vi "Lockin-4461_Multiple Inputs and Outputs_KH.vi"(8 "stop":bool) -> (3 "Input signal":dbl[][](graph))   [LabVIEW 2013]
uses:
  <vilib>/DAQmx/write.llb/DAQmx Write (Analog 1D Wfm NChan NSamp).vi
  DAQ-Lockin-SubVI/Lock-in Globles Multiple Inputs and Outputs used with FGV.vi
  DAQ-Lockin-SubVI/Lock-in Globles Multiple Inputs and Outputs.vi
  <vilib>/DAQmx/miscellaneous.llb/DAQmx Fill In Error Info.vi
  Q:/inst/Leiden measurements VIs/IV measurement/Sub VIs/Global Value.vi
  <vilib>/Analysis/NI_AALPro.lvlib
  <vilib>/Analysis/2dsp.llb/Decimate (single shot, DBL).vi
panel:
  out "Data":waveform(dbl)[][](array[waveform])=[[{"t0"=timestamp(0 s since 1904-01-01), "dt"=5.17729651930355e-06, "Y"=array[14350 elements]}, {"t0"=timestamp(0 s since 1904-01-01), "dt"=5.17729651930355e-06, "Y"=array[14350 elements]}], [{"t0"=timestamp(0 s since 1904-01-01), "dt"=5.17729651930355e-06, "Y"=array[14350 elements]}, {"t0"=timestamp(0 s since 1904-01-01), "dt"=5.17729651930355e-06, "Y"=array[14350 elements]}], [{"t0"=timestamp(0 s since 1904-01-01), "dt"=5.17729651930355e-06, "Y"=array[14350 elements]}, {"t0"=timestamp(0 s since 1904-01-01), "dt"=5.17729651930355e-06, "Y"=array[14350 elements]}], [{"t0"=timestamp(0 s since 1904-01-01), "dt"=5.17729651930355e-06, "Y"=array[14350 elements]}, {"t0"=timestamp(0 s since 1904-01-01), "dt"=5.17729651930355e-06, "Y"=array[14350 elements]}]]
  out "phase log":dbl[](array[numeric])=[0.9999999998974775, 0.9999999998974775, 0.9999999998974775, 0.9999999998974775]
  in  "Tab Control 2":T1(tab)=enum."Lock-in Settings"
  in  "max ai rate":i32=200000
  in  "Auto control  max AI rate/ AI block size":bool=TRUE
  in  "AI Buffer Size (s)":i32=10
  in  "AI Block Size":i32=14350
  out "AI Rate":dbl=193151.0 format="%.2f"
  in  "AI Configuration":T2(array[cluster])=[{"AI.Coupling"=10050, "AI.Max"=10.0, "AI.Min"=-10.0, "Input physical channels"="PXI1Slot2/ai0:1"}, {"AI.Coupling"=10050, "AI.Max"=10.0, "AI.Min"=-10.0, "Input physical channels"="PXI1Slot3/ai0:1"}, {"AI.Coupling"=10050, "AI.Max"=10.0, "AI.Min"=-10.0, "Input physical channels"="PXI1Slot5/ai0:1"}, {"AI.Coupling"=10050, "AI.Max"=10.0, "AI.Min"=-10.0, "Input physical channels"="PXI1Slot6/ai0:1"}] {"AI.Coupling" items=["AC"=10045, "DC"=10050, "GND"=10066]}
  in  "AO Configuration":T3(array[cluster])=[{"Output physical channels"="PXI1Slot2/ao0:1", "AO. Max"=0.1, "AO.Min"=-0.1}, {"Output physical channels"="PXI1Slot3/ao0:1", "AO. Max"=0.25, "AO.Min"=-0.25}, {"Output physical channels"="PXI1Slot5/ao0:1", "AO. Max"=0.1, "AO.Min"=-0.1}, {"Output physical channels"="PXI1Slot6/ao0:1", "AO. Max"=0.1, "AO.Min"=-0.1}]
  in  "OSC Configuration":T4(array[cluster])=[[{"Signal Type"=enum."Sine Wave", "DC"=0.0, "Amplitude"=0.0, "frequency"=13.46, "Phase"=0.0}, {"Signal Type"=enum."Sine Wave", "DC"=0.0, "Amplitude"=0.0005, "frequency"=13.46, "Phase"=0.0}], [{"Signal Type"=enum."Sine Wave", "DC"=0.0, "Amplitude"=0.0, "frequency"=13.46, "Phase"=0.0}, {"Signal Type"=enum."Sine Wave", "DC"=0.0, "Amplitude"=0.0, "frequency"=13.46, "Phase"=0.0}], [{"Signal Type"=enum."Sine Wave", "DC"=0.0, "Amplitude"=0.0, "frequency"=13.46, "Phase"=0.0}, {"Signal Type"=enum."Sine Wave", "DC"=0.0, "Amplitude"=0.0, "frequency"=13.46, "Phase"=0.0}], [{"Signal Type"=enum."Sine Wave", "DC"=-0.0467, "Amplitude"=0.0, "frequency"=13.46, "Phase"=0.0}, {"Signal Type"=enum."Sine Wave", "DC"=0.0, "Amplitude"=0.0, "frequency"=13.46, "Phase"=0.0}]] {"frequency" step=0.001 format="%.3p"; "Amplitude" format="%0.2p"; "DC" min=-0.99 max=0.99 format="%.2p"}
  in  "Phase&Tc":T5(array[cluster])=[{"Phase"=0.0, "Time constant"=0.5, "Set Tc"=FALSE, "Autophase"=FALSE, "Order"=0.0}, {"Phase"=0.0, "Time constant"=0.5, "Set Tc"=FALSE, "Autophase"=FALSE, "Order"=0.0}, {"Phase"=0.0, "Time constant"=0.5, "Set Tc"=FALSE, "Autophase"=FALSE, "Order"=0.0}, {"Phase"=0.0, "Time constant"=0.5, "Set Tc"=FALSE, "Autophase"=FALSE, "Order"=0.0}, {"Phase"=0.0, "Time constant"=0.5, "Set Tc"=FALSE, "Autophase"=FALSE, "Order"=0.0}, {"Phase"=0.0, "Time constant"=0.5, "Set Tc"=FALSE, "Autophase"=FALSE, "Order"=0.0}, {"Phase"=0.0, "Time constant"=0.5, "Set Tc"=FALSE, "Autophase"=FALSE, "Order"=0.0}, {"Phase"=0.0, "Time constant"=0.5, "Set Tc"=FALSE, "Autophase"=FALSE, "Order"=0.0}] {"Phase" min=0.0 max=360.0 scale=0.0..360.0}
  out "Gain":dbl[](array[numeric])=[0.001, 2e-08, 0.001, 0.001, 0.001, 2e-08]
  out "Display 2":string="-189.706780      pA"
  out "Display 1":string="-  1.195069      nA"
  in  "Remote":bool=TRUE
  in  "Display":u16(ring) items=["X and Y", "R and Theta"]
  out "Results":dbl[][](array[numeric])=[[0.0009525094408010766, 3.177938793839466e-05, 0.0009530394348152224, 1.910899317245332], [-0.05975347202365848, -0.009485339009678177, 0.060501645225652, -170.98005941712123], [-3.4755069590434e-06, 9.053140207140873e-07, 3.591481880569719e-06, 165.3998106146712], [0.3512155559510749, -0.06667061103568536, 0.3574875342132845, -10.748465433064244], [0.014508685424842276, -0.002760839766845655, 0.014769028030822714, -10.773934547991182], [0.017218857649450085, -0.002713178173891731, 0.017431305015841704, -8.954481243481103], [-1.0027706515450597e-06, 6.692232605674919e-07, 1.2055740342611434e-06, 146.2818764335927], [-1.3255838707835008e-06, -9.034329256038387e-07, 1.6041707046154658e-06, -145.72416746774206]]
  out "Backlog":u8(slide) scale=0.0..100.0
  out "Sampling information":cluster{"Fs":dbl, "#s":dbl}[](array[cluster])=[{"Fs"=193151.0, "#s"=14350.0}, {"Fs"=193151.0, "#s"=14350.0}, {"Fs"=193151.0, "#s"=14350.0}, {"Fs"=193151.0, "#s"=14350.0}]
  out "AO Task":refnum<k21>[](array[refnum])
  out "AI task":refnum<k21>[](array[refnum])
  out "Signal":dbl[][](array[numeric])
  in  "Tab Control":T6(tab)=enum."Input signals"
  in  "Lockin Display A":i16(slide)=4 scale=1.0..18.0
  out "Display X (or R) A":dbl[](graph)=[0.0003515597766155211, 0.0003507181675748926, 0.00035141371795365553, 0.0003511676429896116, 0.00035187230028368424, 0.00035142951363845783, 0.00035200218342147584, 0.0003516475669745772, 0.0003513264804061819, 0.0003512466291338144, 0.00035057064868592705, 0.0003509796679868739, 0.0003503537452691344, 0.00035135722504198624, 0.0003499281739531895, 0.00035086727974118317, 0.00035123877543565506, 0.00035105622304100427, 0.00035125795255371527, 0.00035135096570343606, 0.00035150903711195496, 0.0003505963637110228, 0.00035169258826266966, 0.00035039322315619063, 0.00035053162210950205, 0.00034979480515196903, 0.00035116833497217555, 0.00035144449100699994, 0.0003510879884516026, 0.00035159349196440626, 0.0003508268451218459, 0.0003511494372195583, 0.0003501864505254134, 0.00035068434585759, 0.0003499157469483272, 0.00035133561940496534, 0.0003501980965627419, 0.0003508062229105727, 0.0003512488754734741, 0.00035101108207568276, 0.000350758527959875, 0.0003505205072637121, 0.0003508151287793871, 0.0003508447380896511, 0.0003507555783012489, 0.0003502437335620398, 0.00035109131124810123, 0.0003498450741887054, 0.00035085670677781735, 0.00034947118732054223, 0.0003511126940251815, 0.0003498712344731183, 0.00035107848043918404, 0.00035092762190149656, 0.00035131019104293144, 0.00035117278992843757, 0.00035060771724494964, 0.00035097354822363525, 0.00034979186802935094, 0.0003511746212457802, 0.0003504305912612818, 0.0003514156401972867, 0.0003503117115571819, 0.0003512893859642446, 0.0003509935260745274, 0.0003513343838004985, 0.00035176841277986657, 0.0003515970316337863, 0.0003513166742771524, 0.00035104054487817416, 0.0003513553972404074, 0.0003509590909684851, 0.00035237906837522605, 0.00034999762062152867, 0.00035101065218240423, 0.0003504366384126203, 0.00035118217997485036, 0.00035142807787819834, 0.00035048373763264237, 0.00035091253545080304, 0.00035015216674575555, 0.00035129179836784774, 0.00035001054715737636, 0.0003513927563841236, 0.0003506721750452684, 0.00035171243027286867, 0.0003514132808403294, 0.00035144774997313054, 0.00035154044709008854, 0.0003519234717441954, 0.0003516730726749858, 0.0003510679416845872, 0.00035125236026625956, 0.0003506717477152614, 0.00035179090850881385, 0.00035059443995565375, 0.0003512356648576366, 0.00035099014639157884, 0.00035160877389527615, 0.0003511922254044786, 0.0003522473208559999, 0.000351701222721286, 0.00035138480038931065, 0.0003513741316379797, 0.0003514851249003675, 0.00035153133788109374, 0.00035099743725480883, 0.0003517112066303713, 0.00035087507155982204, 0.0003514136294778693, 0.00035113141545342375, 0.0003516959886248813, 0.00035089134479069386, 0.00035195932575444284, 0.0003510852464980746, 0.00035095112846043197, 0.00035142787266349444, 0.00035033572449709563, 0.0003518389763278957, 0.0003509974314077956, 0.0003521376695816606, 0.0003512642342070748, 0.00035127618489995405, 0.0003514483445065015, 0.00035163795610624693, 0.00035111410128884024, 0.0003509321167631999, 0.0003510796360339337, 0.0003503292989579528, 0.00035156402647202597, 0.0003512873517971787, 0.00035157967118798955, 0.0003510116552725674, 0.00035141232666041183, 0.00035107492263834197, 0.0003512565883348785, 0.0003508476519342546, 0.00035108010765180813, 0.0003516328893962722, 0.00035126967501414075, 0.00035163302601165687, 0.0003503689014483799, 0.00035132816396016856, 0.00035068072793987285, 0.00035165998148334955, 0.0003506716705224395, 0.00035129129082704685, 0.0003506971941344991, 0.000350963932032198, 0.00035118513223693614, 0.00035074827788279046, 0.0003510020040280428, 0.0003504848068533489, 0.0003513321853419367, 0.0003503106012231704, 0.00035095822008976673, 0.0003502387857211528, 0.00035109477850426885, 0.0003507864147016284, 0.00035140137858089053, 0.0003514994969105284, 0.0003513918557124627, 0.0003513696821528527, 0.0003508483346289989, 0.0003515212484504822, 0.0003510208186503463, 0.00035172200150656446, 0.00035110641441137973, 0.00035150387093385414, 0.000351046214234429, 0.0003512959219150425, 0.00035191226359241245, 0.0003519236956018965, 0.0003521320087141144, 0.00035099481829272187, 0.00035189540980659097, 0.00035122584644459046, 0.00035158482485956113, 0.0003502803891156385, 0.00035140356164375307, 0.0003509192077086382, 0.0003516851651443288, 0.00035113340325199413, 0.0003512155559510749, 0.0003512258338077835, 0.0003520237023195563, 0.00035088778042110256, 0.00035164083859914543, 0.0003511937863128998, 0.0003518097746241161, 0.0003512714055365024, 0.000352054622085523, 0.0003513780489555605, 0.0003520135769537603, 0.00035157613181737254, 0.0003514540449784146, 0.00035148596975263194, 0.00035058490211263083, 0.0003514386933989605, 0.0003509759320918032]
  out "Display Y (or Theta) A":dbl[](graph)=[-6.733399539668474e-05, -6.542411496845478e-05, -6.796694874685229e-05, -6.507135674382902e-05, -6.76731893269279e-05, -6.432724937539189e-05, -6.686858480018215e-05, -6.439302698787755e-05, -6.743074524483553e-05, -6.5540559290562e-05, -6.769912727311773e-05, -6.675855899422707e-05, -6.556455830757394e-05, -6.791926016049456e-05, -6.499870275650685e-05, -6.76094096444829e-05, -6.409372415827203e-05, -6.690358743848511e-05, -6.376319395976735e-05, -6.661678688045064e-05, -6.475221640770524e-05, -6.767037729114109e-05, -6.65568517718371e-05, -6.61078983653106e-05, -6.72090065494324e-05, -6.491767883192775e-05, -6.840639245595013e-05, -6.446292181235111e-05, -6.733865135996714e-05, -6.40653784901512e-05, -6.70766205814384e-05, -6.448431014524983e-05, -6.721244620921082e-05, -6.59878655486392e-05, -6.692322551150028e-05, -6.69019264583306e-05, -6.53521862403277e-05, -6.794558923933263e-05, -6.499376607325872e-05, -6.696965991750598e-05, -6.461599929467364e-05, -6.687775724991745e-05, -6.35960014145792e-05, -6.71748832581576e-05, -6.492398900048032e-05, -6.746798157246069e-05, -6.634689247733003e-05, -6.592248825579343e-05, -6.76983125588508e-05, -6.466202421410609e-05, -6.750345332833928e-05, -6.450271804110632e-05, -6.73820213196671e-05, -6.398878990855814e-05, -6.699882608984017e-05, -6.499280498169577e-05, -6.738425010553764e-05, -6.660128249440328e-05, -6.641623559943719e-05, -6.741839015150833e-05, -6.490399197802229e-05, -6.807262637843706e-05, -6.461095964170923e-05, -6.741693933791136e-05, -6.396241139824065e-05, -6.68953533836962e-05, -6.437486412654718e-05, -6.719672530343625e-05, -6.601025951582242e-05, -6.755243507643756e-05, -6.683904754234452e-05, -6.581328668735525e-05, -6.7956730495926e-05, -6.454210702322087e-05, -6.700846714162137e-05, -6.487036358948187e-05, -6.717145047610366e-05, -6.394657730710213e-05, -6.721398561579939e-05, -6.542844878392274e-05, -6.72242800275423e-05, -6.601836591155777e-05, -6.679640312152599e-05, -6.724964008795247e-05, -6.524389201445212e-05, -6.81709788892876e-05, -6.504870506524659e-05, -6.716417310946288e-05, -6.469364606167295e-05, -6.64118927639841e-05, -6.428422401809015e-05, -6.726075100677492e-05, -6.602001398773281e-05, -6.684946783051746e-05, -6.665356018961591e-05, -6.559302821306713e-05, -6.823961541895857e-05, -6.489902378019219e-05, -6.747231633806965e-05, -6.460461787722171e-05, -6.739619325891061e-05, -6.42568749063365e-05, -6.728357578332122e-05, -6.572581320455293e-05, -6.733133575279844e-05, -6.745384605205556e-05, -6.654768580556922e-05, -6.752884945881219e-05, -6.516474446690376e-05, -6.800609459823608e-05, -6.47878614014136e-05, -6.730160658797204e-05, -6.420250070636625e-05, -6.676581343835398e-05, -6.447454426249553e-05, -6.739644425949934e-05, -6.633928104016707e-05, -6.668506011610336e-05, -6.704708770176857e-05, -6.518924517552728e-05, -6.80110716513718e-05, -6.449044290923919e-05, -6.713463098761624e-05, -6.431427908560736e-05, -6.666702370071547e-05, -6.380160055564429e-05, -6.69295226583365e-05, -6.559831844106169e-05, -6.733302905782082e-05, -6.676258268638944e-05, -6.581664753168712e-05, -6.791627178025961e-05, -6.483985086130437e-05, -6.771582429628417e-05, -6.456692771022534e-05, -6.710554331363558e-05, -6.416205680544463e-05, -6.721382973122853e-05, -6.497521331755278e-05, -6.762221774081424e-05, -6.644148745970977e-05, -6.650204706057299e-05, -6.779409446006897e-05, -6.513429971844772e-05, -6.716283035881229e-05, -6.500520220536936e-05, -6.748818593189037e-05, -6.375021526081944e-05, -6.679304519274533e-05, -6.44009832356367e-05, -6.697029619860621e-05, -6.614507717764695e-05, -6.675045380090485e-05, -6.699368958403159e-05, -6.540977419016514e-05, -6.751824094235534e-05, -6.497224203386006e-05, -6.747996187391402e-05, -6.445371747351958e-05, -6.694216412544935e-05, -6.39145549472495e-05, -6.67208337122775e-05, -6.499887641961741e-05, -6.75636406906266e-05, -6.646187561893783e-05, -6.6422353672184e-05, -6.774188283466967e-05, -6.49718493653088e-05, -6.774060340062207e-05, -6.447729538855726e-05, -6.7276329542447e-05, -6.45413468122233e-05, -6.725796598454556e-05, -6.43215545435326e-05, -6.710426281533913e-05, -6.640793922515245e-05, -6.688725807556598e-05, -6.702595030422637e-05, -6.555532275656158e-05, -6.775334049196785e-05, -6.485489689304207e-05, -6.778283710493148e-05, -6.47406497658257e-05, -6.667061103568536e-05, -6.71178176816977e-05, -6.545036016336727e-05, -6.758648874374465e-05, -6.648186107488955e-05, -6.564351224820166e-05, -6.726344507999936e-05, -6.562770441403993e-05, -6.793015780847218e-05, -6.469220243177453e-05, -6.740767551952607e-05, -6.44720529171589e-05, -6.682838905210087e-05, -6.483406975990464e-05, -6.710332224721377e-05, -6.629467593853179e-05, -6.657765389063085e-05]
  in  "Lockin Display B":i16(slide)=2 scale=1.0..18.0
  out "Display X (or R) B":dbl[](graph)=[-5.973805372889475e-05, -5.997769367534496e-05, -5.9708287795621276e-05, -5.984678440204925e-05, -5.96020365229781e-05, -5.988348783189898e-05, -5.955411213886451e-05, -5.966114639955685e-05, -5.967736545809988e-05, -5.9802807819580876e-05, -6.032026368325063e-05, -6.001689267914097e-05, -6.003410657029983e-05, -5.977018506520212e-05, -6.0340734789310514e-05, -5.993900458976907e-05, -5.9820041306625844e-05, -5.9903553468692154e-05, -5.9952134877729026e-05, -5.979215433879489e-05, -5.979055625375601e-05, -5.987510686924956e-05, -5.9788578934364e-05, -6.0192416860962845e-05, -5.993209011456587e-05, -6.033457353599281e-05, -5.971909732158195e-05, -5.996045369372309e-05, -5.974130155444159e-05, -5.9706581716911424e-05, -5.9853671695556514e-05, -6.002410357943405e-05, -6.028871998471762e-05, -5.9785222068695644e-05, -6.03349447986027e-05, -5.984123442332923e-05, -6.020997572427012e-05, -5.995797702359279e-05, -5.979901045458895e-05, -5.986307354486177e-05, -5.98177204998572e-05, -5.993627036242485e-05, -5.999707011009087e-05, -5.997537248897983e-05, -6.0275622555272004e-05, -5.998718512494211e-05, -6.0025859867444536e-05, -6.028432464437489e-05, -5.980624038568292e-05, -6.025710548995174e-05, -5.9918096477315704e-05, -6.00761402076088e-05, -5.981242212931597e-05, -5.996635489034251e-05, -5.961826607421154e-05, -5.985414477478984e-05, -6.0063476407074825e-05, -6.010302629401186e-05, -6.026166887569885e-05, -5.967151917856465e-05, -6.018706695966701e-05, -5.9636349964672865e-05, -6.011958688712653e-05, -5.977560321458471e-05, -5.988776705568878e-05, -5.977496924007715e-05, -5.9581733793994986e-05, -5.957529493552923e-05, -5.968823353723063e-05, -5.986788099315147e-05, -5.973198851548897e-05, -6.001154219913467e-05, -5.91698731876615e-05, -6.0154657926692944e-05, -5.962357974201017e-05, -6.0119914876982445e-05, -5.98418042765305e-05, -5.966781036322989e-05, -6.007055241654932e-05, -5.977139212057935e-05, -5.99633957162437e-05, -5.972348085326211e-05, -6.0018193608286176e-05, -5.9790857121652925e-05, -5.9931625506878436e-05, -5.94844330711744e-05, -5.9986973718200476e-05, -5.9767122422151896e-05, -5.952282668641666e-05, -5.962989054624437e-05, -5.954335861112378e-05, -5.985757597779662e-05, -5.9899408226975814e-05, -5.989722350926432e-05, -5.955987204612377e-05, -6.007759278589658e-05, -5.965609768633246e-05, -5.987720054549058e-05, -5.956473916807613e-05, -5.9726527069550545e-05, -5.9332614966000636e-05, -5.9464756469964765e-05, -5.96012958531051e-05, -5.9766885184994385e-05, -5.974761549750783e-05, -5.950143497831813e-05, -5.9792686364383365e-05, -5.934483722266e-05, -6.008374831181307e-05, -5.944823582629368e-05, -5.9548780520340945e-05, -5.965224668704047e-05, -5.9919961480994526e-05, -5.954592619442524e-05, -5.9923241555092845e-05, -5.984879370896418e-05, -5.967338877703454e-05, -6.0046522311407315e-05, -5.956301238222821e-05, -5.9980996077878475e-05, -5.915640181989461e-05, -5.9672842983131156e-05, -5.955409158466315e-05, -5.9669841807045967e-05, -5.938651343510987e-05, -5.988305753970675e-05, -5.9786820620838744e-05, -5.9815068956163915e-05, -6.019429820706566e-05, -5.960804114856816e-05, -5.985252073379312e-05, -5.9395944114833624e-05, -6.003627751220466e-05, -5.938654131424103e-05, -6.006609300669626e-05, -5.952810733038762e-05, -6.007816486380681e-05, -5.9939317080817105e-05, -5.969907931438443e-05, -6.018611821347548e-05, -5.9591701319973753e-05, -6.012708358934569e-05, -5.965802693027772e-05, -5.9883610899726214e-05, -5.941512185906086e-05, -6.008393935063718e-05, -5.971205707747965e-05, -5.9825812366495034e-05, -5.982134839858187e-05, -5.990673551573905e-05, -5.991075453489442e-05, -5.980745152168868e-05, -6.016420809204294e-05, -5.9866112875718205e-05, -5.994862774833857e-05, -5.963278108763234e-05, -6.019497134354614e-05, -5.967916947543666e-05, -6.001763722947105e-05, -5.987197709186515e-05, -5.935733819858279e-05, -5.986783223760929e-05, -6.005067229334361e-05, -6.006190323740792e-05, -5.94483748789149e-05, -5.9816898924531726e-05, -5.9490861689937646e-05, -5.966154589050948e-05, -5.959148517379623e-05, -5.967660993779421e-05, -5.968571170388341e-05, -5.9487283620622405e-05, -5.938567148253452e-05, -5.9644953885369794e-05, -5.986165657982996e-05, -5.943676086750176e-05, -5.960174349530741e-05, -5.965486357155142e-05, -5.9995280805136567e-05, -5.962821603489821e-05, -6.0003638585563e-05, -5.958692938826757e-05, -6.000685979841328e-05, -5.9753472023658484e-05, -5.979998802096852e-05, -5.9698506548474515e-05, -5.9846945821246745e-05, -5.963523327520546e-05, -5.9901187291550265e-05, -5.941349662406738e-05, -5.983522571052821e-05, -5.961196352889655e-05, -5.964719105393711e-05, -5.9455369335570684e-05, -5.9850548883224846e-05, -5.9687681880990575e-05, -5.9741782783296065e-05, -6.004274754126064e-05, -5.9772984300660404e-05, -5.965611478541512e-05]
  out "Display Y (or Theta) B":dbl[](graph)=[-8.958270649644575e-06, -9.079174417097126e-06, -9.722869303426089e-06, -8.670926842445195e-06, -9.798896241530504e-06, -8.578655474373097e-06, -9.839033227838285e-06, -8.725745473856126e-06, -1.0110185040810307e-05, -8.88178957036905e-06, -1.0068917475673968e-05, -9.152677048848094e-06, -8.872108126948592e-06, -9.615107554782487e-06, -8.542521794571126e-06, -9.734611314161527e-06, -8.62277737722622e-06, -9.72189703622162e-06, -8.347977989417005e-06, -9.826850753961157e-06, -8.765135719942297e-06, -1.0384261380866108e-05, -9.283496688400475e-06, -9.298531240255045e-06, -9.131942536820838e-06, -8.834486063190045e-06, -1.0002259864072125e-05, -8.605747988725545e-06, -9.718976848430474e-06, -8.616023269702668e-06, -9.775399440134439e-06, -8.694800931184639e-06, -1.0164140966682503e-05, -8.991971356660822e-06, -1.008925932009518e-05, -9.135704007433286e-06, -9.075412639207577e-06, -9.768029366199697e-06, -8.572138210499408e-06, -9.54652028693435e-06, -8.297060155110535e-06, -9.836618324290022e-06, -8.430082903824597e-06, -1.0142883387518154e-05, -8.941978388845142e-06, -1.01850937594548e-05, -8.731222939193217e-06, -9.221840410817993e-06, -9.432758625652156e-06, -8.64474181423124e-06, -9.47902609950266e-06, -8.602368720920302e-06, -9.6402357444777e-06, -8.508673879951827e-06, -1.0171813153030253e-05, -8.762585465396693e-06, -1.0143747737022767e-05, -9.075082749076048e-06, -9.398764904572573e-06, -9.307073418577166e-06, -8.793098488533298e-06, -9.637112070416567e-06, -8.507505668559803e-06, -9.476377379412959e-06, -8.348372976729366e-06, -9.609504624542375e-06, -8.492413951458167e-06, -1.0187132012055195e-05, -9.247097418557014e-06, -1.0008237209153778e-05, -9.110005111830295e-06, -8.868365137084955e-06, -9.497753879190364e-06, -8.54691807040817e-06, -9.492940438086256e-06, -8.86534519730119e-06, -9.75061426619826e-06, -8.22996966160815e-06, -9.959245472180723e-06, -9.080959296505907e-06, -9.946242551003338e-06, -8.999064761142276e-06, -9.544634912731375e-06, -9.333691047585492e-06, -8.71461480093321e-06, -9.749628892132326e-06, -8.696242663003042e-06, -9.571537831850369e-06, -8.665272678702301e-06, -9.790645025081464e-06, -8.590382009269797e-06, -1.0054380465985972e-05, -9.143736631964047e-06, -9.83766237226238e-06, -8.963523918085618e-06, -9.023864930532281e-06, -9.775546338514358e-06, -8.743072840756056e-06, -9.750048748115978e-06, -8.63249001811124e-06, -9.779209409133608e-06, -8.555540235636452e-06, -1.0147771789992131e-05, -9.085662280344776e-06, -9.948357858388622e-06, -9.236666490990091e-06, -9.405014940831864e-06, -9.556314415693313e-06, -8.978396257346734e-06, -9.660193811970222e-06, -8.591888505258487e-06, -9.819894369143736e-06, -8.499382068804003e-06, -9.889218466287092e-06, -8.560910632236936e-06, -1.018883863587036e-05, -9.189988665614938e-06, -9.642383360284503e-06, -9.356225736166237e-06, -8.949099957359457e-06, -9.556605113224137e-06, -8.449679998334245e-06, -9.558118590243917e-06, -8.417513167464567e-06, -9.828861338705494e-06, -8.29071798884531e-06, -1.007556270817022e-05, -9.049851316193156e-06, -9.870069569853969e-06, -9.188054666626924e-06, -9.014512165071601e-06, -9.426128868088451e-06, -8.800537418901013e-06, -9.599330459942152e-06, -8.489523225135791e-06, -9.757050945790948e-06, -8.614032410791086e-06, -1.0108554297528621e-05, -8.833190731386632e-06, -1.0317624573594027e-05, -9.01342212907643e-06, -9.453674652460764e-06, -9.463587844990278e-06, -8.86880836495292e-06, -9.551751716676205e-06, -8.474263724880662e-06, -9.477246756111029e-06, -8.422698325464234e-06, -9.66171158313459e-06, -8.660761021498567e-06, -9.980759525866703e-06, -8.874944766903318e-06, -9.89170445476312e-06, -8.909652219119875e-06, -8.927901827996496e-06, -9.532741250467193e-06, -8.769219635249499e-06, -9.45489494261844e-06, -8.459543432736222e-06, -9.517236911159184e-06, -8.386576048857434e-06, -9.943702053335803e-06, -8.689970534079697e-06, -1.0221696926853864e-05, -8.95026150178313e-06, -9.411851276772798e-06, -9.646423426510309e-06, -8.88955144628328e-06, -9.602816172952274e-06, -8.254310166427626e-06, -9.714813429673415e-06, -8.609274632068607e-06, -9.980947496577697e-06, -8.613011646308823e-06, -9.926523035995543e-06, -9.437162149941353e-06, -9.85730084147906e-06, -9.056211093468829e-06, -9.134490532887283e-06, -9.547055813053063e-06, -8.542618511288604e-06, -9.588512074352255e-06, -8.723779851578767e-06, -9.485339009678177e-06, -9.927192587986094e-06, -9.027493998535825e-06, -1.0154050329471879e-05, -8.942734822055541e-06, -8.99875305703814e-06, -9.23104061835275e-06, -8.902905742370081e-06, -9.68735374617075e-06, -8.481819818693765e-06, -9.612193271817266e-06, -8.588515380675596e-06, -9.910536092220234e-06, -8.881932812600387e-06, -1.024879999065798e-05, -9.087511987205371e-06, -9.336166971779956e-06]
  in  "Lockin Display C":i16(slide)=3 scale=1.0..18.0
  out "Display X (or R) C":dbl[](graph)=[-4.8668293250196435e-09, -3.745115284293864e-09, -3.378579300703624e-09, -3.962538699481019e-09, -3.7052129160729895e-09, -3.7002490402748057e-09, -4.98089238947947e-09, -3.8703191594580585e-09, -2.8878815784256017e-09, -4.294393565461846e-09, -3.460819365757349e-09, -3.572068148924036e-09, -3.973202623999354e-09, -3.426934288130705e-09, -4.9065826450738035e-09, -3.6312644598121367e-09, -3.868182699065086e-09, -3.802259105591664e-09, -4.1017027350523075e-09, -2.3899421106473476e-09, -3.4373213909624433e-09, -4.3395506609927135e-09, -2.639102842602597e-09, -4.26495140716537e-09, -4.264732303883781e-09, -5.1934190246123324e-09, -3.9694818894077045e-09, -4.078638241864219e-09, -5.609993051780682e-09, -4.545204199496178e-09, -3.181332786031654e-09, -3.0786977982040526e-09, -3.531353714412713e-09, -3.845660743926098e-09, -3.1270362531041545e-09, -3.3649353207679793e-09, -3.892936060852318e-09, -5.327095540435721e-09, -2.859172584498669e-09, -4.08564429698212e-09, -4.6245041783795585e-09, -3.96876992651159e-09, -4.912378771606807e-09, -3.9575866665511424e-09, -5.4717768680449005e-09, -4.093163234729508e-09, -4.061455678483012e-09, -3.854586999323003e-09, -3.6971380166764782e-09, -2.7792135887819638e-09, -3.8167401853553656e-09, -1.636876859605488e-09, -3.6533415669137195e-09, -4.957159249294414e-09, -2.935545278103778e-09, -4.167214373396586e-09, -3.7966739320631305e-09, -3.846169296100357e-09, -3.6080210517721625e-09, -3.5108425256632506e-09, -4.13911824348043e-09, -2.957824944582016e-09, -3.6427320301477585e-09, -3.648726219082018e-09, -4.077859370416953e-09, -2.3823897023614617e-09, -3.903617522836711e-09, -3.9487103772262865e-09, -3.0519177635676944e-09, -3.79261977695756e-09, -5.249247334263507e-09, -3.7339534392611515e-09, -4.107738112546451e-09, -3.52630924701912e-09, -4.338867825020414e-09, -3.1210439333613185e-09, -3.2947613659106337e-09, -5.663049786573686e-09, -3.0645468568072034e-09, -6.100387585007984e-09, -3.1326265185584843e-09, -2.713971324808483e-09, -4.8344399051411294e-09, -2.779814970922091e-09, -3.1387832858016756e-09, -3.5995134187258946e-09, -4.019447183960172e-09, -4.3421720781246565e-09, -4.42442598534967e-09, -2.0343195493401075e-09, -3.3280813962148666e-09, -4.857914656153474e-09, -1.9553510903220776e-09, -4.1813474548531525e-09, -3.866313724881681e-09, -2.1623950794469502e-09, -3.854852775185502e-09, -3.869096709501723e-09, -3.6817272437978513e-09, -4.453098468921171e-09, -3.995188216635368e-09, -5.290481140158009e-09, -4.371378358051492e-09, -3.429876252324654e-09, -4.287891116944586e-09, -3.6037342414452737e-09, -3.594911646344261e-09, -4.084912754180051e-09, -2.952177900736285e-09, -3.1760349575051898e-09, -4.9482189948013884e-09, -2.5930147890330783e-09, -4.703665970223814e-09, -4.927494827780477e-09, -4.501667206106983e-09, -2.4962299417468718e-09, -4.47618116049368e-09, -4.985769548834164e-09, -3.0195125349603775e-09, -3.4917032552159702e-09, -3.808937658076576e-09, -3.985372148913932e-09, -3.340467508204991e-09, -3.468800615806591e-09, -3.112411475019484e-09, -4.85493783805854e-09, -2.95185572361082e-09, -3.773064773778177e-09, -3.916303288000469e-09, -3.532422785377317e-09, -3.859141581207644e-09, -3.7008884425477863e-09, -4.1002784097759445e-09, -2.7514323389457215e-09, -2.3514239819218798e-09, -3.872816477539419e-09, -3.5780586835082263e-09, -3.81955963330902e-09, -2.4293102054569633e-09, -3.382540400396762e-09, -5.5428180977782255e-09, -2.7795096479751987e-09, -3.804222999220076e-09, -3.4803551604071215e-09, -5.234153587505983e-09, -2.458659364856988e-09, -3.147526362885383e-09, -3.4236646233945987e-09, -3.241678157094595e-09, -3.947836838802674e-09, -3.998694389047356e-09, -3.8966170731906045e-09, -3.2634453310819047e-09, -3.360764287977601e-09, -3.858276387773567e-09, -2.730545274800396e-09, -3.734633224357905e-09, -3.925669797939688e-09, -4.089059228871761e-09, -3.1167948214178144e-09, -4.960389927626379e-09, -3.943981322171711e-09, -4.449291327128986e-09, -3.1883376357130596e-09, -3.3067072057954027e-09, -3.3189371777593753e-09, -4.01735625078221e-09, -4.341033778514668e-09, -3.5647126071332782e-09, -3.1771707793763404e-09, -4.547628482305568e-09, -4.1274692424744e-09, -3.847369312070051e-09, -4.2240684565703186e-09, -4.9666111872453606e-09, -3.5189017076481715e-09, -3.715881166405545e-09, -2.9541048588757674e-09, -3.7376705439394596e-09, -3.363931270423648e-09, -4.990406950834843e-09, -3.783561513877033e-09, -4.100387183486353e-09, -3.4755069590433998e-09, -2.0587973667347604e-09, -3.747377938878194e-09, -5.047638105098522e-09, -3.444693785255246e-09, -4.257325911453854e-09, -2.9478372104314067e-09, -4.8693771424641264e-09, -2.8340474279218866e-09, -3.634779856606349e-09, -3.1785815856409e-09, -4.8383990187620576e-09, -4.803717448877167e-09, -4.261576832842807e-09, -2.820953059028035e-09, -2.967748740261674e-09, -4.470017681501436e-09]
  out "Display Y (or Theta) C":dbl[](graph)=[1.162601126425967e-09, -1.1048492330906777e-10, 1.7034370463595466e-09, 1.227552491294126e-09, 1.1347106133830338e-09, 1.1671830886335785e-09, 1.6927599366013312e-09, 2.03804612323238e-09, 2.440980679995142e-10, 2.844269383862327e-09, 2.2535472729773546e-10, 1.0382143914054814e-09, -5.106420747080373e-10, 7.245646925706077e-10, 2.5379437220700634e-09, 2.7522957282572883e-09, 1.7615504978887316e-09, 1.0910805838443012e-09, 5.80086448264603e-10, 5.243607188795422e-10, 2.656108918703469e-09, 3.835670989666289e-10, 5.253438645389102e-10, 2.356336299624039e-10, 1.5802950683625581e-09, 6.122772119933944e-10, 1.918721050974528e-09, 1.6779694119770094e-09, 2.2566803050548513e-09, 6.032256583276967e-10, 1.1888145636897593e-09, 1.722199890225765e-09, 1.350790537371745e-09, 5.605654981866342e-10, 2.517973696938616e-10, 3.261718237136838e-09, 1.2902919354996673e-10, 1.1514276353018522e-09, 1.136745252005257e-09, 4.401878109841974e-10, -2.9702967851871836e-11, 1.041007748859096e-09, 9.266456242864077e-10, 1.0927524248642774e-09, 6.214157561010142e-10, 1.6049954189162906e-09, 1.5055328962593048e-09, -3.8737736516234496e-10, 2.750717324146772e-09, 1.990333539307104e-09, 2.1640357576029394e-09, 1.134319865647604e-09, 2.057697918465208e-09, 1.630534369627498e-09, 1.8595093581473553e-09, 2.6035142992563592e-09, 4.3932972364002686e-10, 1.4850494865211682e-09, 1.2177648083059968e-09, 8.241532895772667e-10, 1.052510465576346e-09, 2.844298052433484e-09, 1.0497759585199982e-09, 1.8748501742630355e-09, 2.440410809214677e-10, 1.1760580599292533e-09, 2.2106861530790015e-09, 1.944116883252444e-09, 3.1155663701856266e-10, -2.6065372346242703e-10, 3.9623653989711296e-10, -5.608877612116372e-10, 1.6522809093940316e-09, 2.3673818368562105e-10, 1.032980330302756e-09, 9.738020388136405e-10, 9.049738556668177e-10, 1.3276249889899394e-09, 1.5628917066366904e-09, 1.1434661538750887e-09, -1.4111843267076968e-09, 2.0464457889505905e-09, 1.1502239291332387e-09, 1.7258071701690818e-09, 2.870316384325903e-10, 1.9470923602157385e-09, 1.1280879856207515e-09, 2.3836815039016263e-09, 1.5382787638613197e-09, -3.5139584116294666e-11, 1.5339775557459824e-09, 3.447629446431663e-10, 1.2314039731938668e-09, 5.628109172323627e-11, 2.73486862512292e-09, 1.447313399369049e-10, 1.6948027186744173e-09, 9.46215019600876e-10, 1.6199491631605202e-09, 1.2125682983718194e-09, 1.7494550240206437e-09, 1.2723350927478245e-09, 1.294274033538532e-09, 2.167234382494876e-09, -3.801690244653738e-10, 1.870610305707888e-09, -1.8855874978149187e-10, 2.8932325164786413e-09, 1.2292553884673413e-09, 2.5023423668819587e-09, 1.0951495754581317e-09, 1.6831995284616958e-09, 9.655697884139497e-10, 6.512569933241963e-10, 1.91386771940341e-09, 1.27817939858807e-09, 1.2913096892076088e-09, 5.816532091176878e-10, 1.4730157460001533e-09, 6.807522347301478e-10, 2.5740800064144563e-09, 4.990614039776123e-10, 1.3207746335717788e-09, 5.194313039533898e-11, 1.326519413687359e-09, 5.868869587408655e-10, 6.701449099930656e-11, 2.779293671403518e-10, 1.1048459849926027e-09, 2.2730451576367575e-09, 5.56830090717463e-10, 1.9135846334161137e-09, -2.4930533074226744e-10, 1.621866264423612e-09, 1.5157709386455977e-09, 2.3689077476706544e-09, 2.604404152139465e-10, 1.3767538209895341e-09, 1.6481775932096413e-09, 7.563164910886242e-10, 2.732254768261487e-09, -9.3044419314283e-10, 2.4195087798867362e-09, -2.767922203295941e-10, 2.404046840007802e-09, 9.589472897058583e-10, 2.954812065406236e-09, -1.780154545786323e-10, 1.4947577045123354e-09, 2.0602202752298724e-11, 4.141191745480916e-10, 8.117608349243262e-10, 1.8151012166052304e-09, 2.074060568998317e-09, 4.233835518114647e-10, 2.5384111737494713e-09, 9.845561685456097e-10, 1.978876362560332e-09, 1.73981547830828e-09, 1.6298902611637085e-09, 1.320745443234922e-09, 1.4376002811712767e-09, 1.3247399753964818e-09, 3.27338698947474e-10, 2.610940156669763e-09, 1.502019986937931e-10, 1.8356378144653108e-09, 1.8452845172917403e-09, 2.300216632032428e-09, 1.3904793422911363e-09, 2.079980448486155e-09, 1.3072196840722395e-09, 2.090911084590946e-09, 9.782994263485832e-10, 1.4723228325857777e-09, 2.1298117823935e-09, 4.6482767363481033e-10, 2.3150822180769145e-09, 8.266352716183207e-10, 1.897992779083837e-09, 1.7488248789075386e-09, 1.5142711964056431e-09, 2.2526201822234644e-09, 9.053140207140873e-10, 1.6728873826394462e-09, 1.7882941434042654e-09, 2.1013305702521744e-09, 2.3257746843917406e-09, -1.246867261662684e-09, 2.027926867834542e-09, -3.1423088829967834e-10, 1.5528140352245746e-09, 1.3041768778855137e-09, 1.7331796632548882e-09, 1.8608207777580392e-09, 3.827610336757765e-10, 1.4146637573937803e-09, 1.5207957427241911e-09, 1.410403109776104e-09, 4.249982867711876e-10]
  in  "Lockin Display D":i16(slide)=4 scale=1.0..18.0
  out "Display X (or R) D":dbl[](graph)=[0.0003515597766155211, 0.0003507181675748926, 0.00035141371795365553, 0.0003511676429896116, 0.00035187230028368424, 0.00035142951363845783, 0.00035200218342147584, 0.0003516475669745772, 0.0003513264804061819, 0.0003512466291338144, 0.00035057064868592705, 0.0003509796679868739, 0.0003503537452691344, 0.00035135722504198624, 0.0003499281739531895, 0.00035086727974118317, 0.00035123877543565506, 0.00035105622304100427, 0.00035125795255371527, 0.00035135096570343606, 0.00035150903711195496, 0.0003505963637110228, 0.00035169258826266966, 0.00035039322315619063, 0.00035053162210950205, 0.00034979480515196903, 0.00035116833497217555, 0.00035144449100699994, 0.0003510879884516026, 0.00035159349196440626, 0.0003508268451218459, 0.0003511494372195583, 0.0003501864505254134, 0.00035068434585759, 0.0003499157469483272, 0.00035133561940496534, 0.0003501980965627419, 0.0003508062229105727, 0.0003512488754734741, 0.00035101108207568276, 0.000350758527959875, 0.0003505205072637121, 0.0003508151287793871, 0.0003508447380896511, 0.0003507555783012489, 0.0003502437335620398, 0.00035109131124810123, 0.0003498450741887054, 0.00035085670677781735, 0.00034947118732054223, 0.0003511126940251815, 0.0003498712344731183, 0.00035107848043918404, 0.00035092762190149656, 0.00035131019104293144, 0.00035117278992843757, 0.00035060771724494964, 0.00035097354822363525, 0.00034979186802935094, 0.0003511746212457802, 0.0003504305912612818, 0.0003514156401972867, 0.0003503117115571819, 0.0003512893859642446, 0.0003509935260745274, 0.0003513343838004985, 0.00035176841277986657, 0.0003515970316337863, 0.0003513166742771524, 0.00035104054487817416, 0.0003513553972404074, 0.0003509590909684851, 0.00035237906837522605, 0.00034999762062152867, 0.00035101065218240423, 0.0003504366384126203, 0.00035118217997485036, 0.00035142807787819834, 0.00035048373763264237, 0.00035091253545080304, 0.00035015216674575555, 0.00035129179836784774, 0.00035001054715737636, 0.0003513927563841236, 0.0003506721750452684, 0.00035171243027286867, 0.0003514132808403294, 0.00035144774997313054, 0.00035154044709008854, 0.0003519234717441954, 0.0003516730726749858, 0.0003510679416845872, 0.00035125236026625956, 0.0003506717477152614, 0.00035179090850881385, 0.00035059443995565375, 0.0003512356648576366, 0.00035099014639157884, 0.00035160877389527615, 0.0003511922254044786, 0.0003522473208559999, 0.000351701222721286, 0.00035138480038931065, 0.0003513741316379797, 0.0003514851249003675, 0.00035153133788109374, 0.00035099743725480883, 0.0003517112066303713, 0.00035087507155982204, 0.0003514136294778693, 0.00035113141545342375, 0.0003516959886248813, 0.00035089134479069386, 0.00035195932575444284, 0.0003510852464980746, 0.00035095112846043197, 0.00035142787266349444, 0.00035033572449709563, 0.0003518389763278957, 0.0003509974314077956, 0.0003521376695816606, 0.0003512642342070748, 0.00035127618489995405, 0.0003514483445065015, 0.00035163795610624693, 0.00035111410128884024, 0.0003509321167631999, 0.0003510796360339337, 0.0003503292989579528, 0.00035156402647202597, 0.0003512873517971787, 0.00035157967118798955, 0.0003510116552725674, 0.00035141232666041183, 0.00035107492263834197, 0.0003512565883348785, 0.0003508476519342546, 0.00035108010765180813, 0.0003516328893962722, 0.00035126967501414075, 0.00035163302601165687, 0.0003503689014483799, 0.00035132816396016856, 0.00035068072793987285, 0.00035165998148334955, 0.0003506716705224395, 0.00035129129082704685, 0.0003506971941344991, 0.000350963932032198, 0.00035118513223693614, 0.00035074827788279046, 0.0003510020040280428, 0.0003504848068533489, 0.0003513321853419367, 0.0003503106012231704, 0.00035095822008976673, 0.0003502387857211528, 0.00035109477850426885, 0.0003507864147016284, 0.00035140137858089053, 0.0003514994969105284, 0.0003513918557124627, 0.0003513696821528527, 0.0003508483346289989, 0.0003515212484504822, 0.0003510208186503463, 0.00035172200150656446, 0.00035110641441137973, 0.00035150387093385414, 0.000351046214234429, 0.0003512959219150425, 0.00035191226359241245, 0.0003519236956018965, 0.0003521320087141144, 0.00035099481829272187, 0.00035189540980659097, 0.00035122584644459046, 0.00035158482485956113, 0.0003502803891156385, 0.00035140356164375307, 0.0003509192077086382, 0.0003516851651443288, 0.00035113340325199413, 0.0003512155559510749, 0.0003512258338077835, 0.0003520237023195563, 0.00035088778042110256, 0.00035164083859914543, 0.0003511937863128998, 0.0003518097746241161, 0.0003512714055365024, 0.000352054622085523, 0.0003513780489555605, 0.0003520135769537603, 0.00035157613181737254, 0.0003514540449784146, 0.00035148596975263194, 0.00035058490211263083, 0.0003514386933989605, 0.0003509759320918032]
  out "Display Y (or Theta) D":dbl[](graph)=[-6.733399539668474e-05, -6.542411496845478e-05, -6.796694874685229e-05, -6.507135674382902e-05, -6.76731893269279e-05, -6.432724937539189e-05, -6.686858480018215e-05, -6.439302698787755e-05, -6.743074524483553e-05, -6.5540559290562e-05, -6.769912727311773e-05, -6.675855899422707e-05, -6.556455830757394e-05, -6.791926016049456e-05, -6.499870275650685e-05, -6.76094096444829e-05, -6.409372415827203e-05, -6.690358743848511e-05, -6.376319395976735e-05, -6.661678688045064e-05, -6.475221640770524e-05, -6.767037729114109e-05, -6.65568517718371e-05, -6.61078983653106e-05, -6.72090065494324e-05, -6.491767883192775e-05, -6.840639245595013e-05, -6.446292181235111e-05, -6.733865135996714e-05, -6.40653784901512e-05, -6.70766205814384e-05, -6.448431014524983e-05, -6.721244620921082e-05, -6.59878655486392e-05, -6.692322551150028e-05, -6.69019264583306e-05, -6.53521862403277e-05, -6.794558923933263e-05, -6.499376607325872e-05, -6.696965991750598e-05, -6.461599929467364e-05, -6.687775724991745e-05, -6.35960014145792e-05, -6.71748832581576e-05, -6.492398900048032e-05, -6.746798157246069e-05, -6.634689247733003e-05, -6.592248825579343e-05, -6.76983125588508e-05, -6.466202421410609e-05, -6.750345332833928e-05, -6.450271804110632e-05, -6.73820213196671e-05, -6.398878990855814e-05, -6.699882608984017e-05, -6.499280498169577e-05, -6.738425010553764e-05, -6.660128249440328e-05, -6.641623559943719e-05, -6.741839015150833e-05, -6.490399197802229e-05, -6.807262637843706e-05, -6.461095964170923e-05, -6.741693933791136e-05, -6.396241139824065e-05, -6.68953533836962e-05, -6.437486412654718e-05, -6.719672530343625e-05, -6.601025951582242e-05, -6.755243507643756e-05, -6.683904754234452e-05, -6.581328668735525e-05, -6.7956730495926e-05, -6.454210702322087e-05, -6.700846714162137e-05, -6.487036358948187e-05, -6.717145047610366e-05, -6.394657730710213e-05, -6.721398561579939e-05, -6.542844878392274e-05, -6.72242800275423e-05, -6.601836591155777e-05, -6.679640312152599e-05, -6.724964008795247e-05, -6.524389201445212e-05, -6.81709788892876e-05, -6.504870506524659e-05, -6.716417310946288e-05, -6.469364606167295e-05, -6.64118927639841e-05, -6.428422401809015e-05, -6.726075100677492e-05, -6.602001398773281e-05, -6.684946783051746e-05, -6.665356018961591e-05, -6.559302821306713e-05, -6.823961541895857e-05, -6.489902378019219e-05, -6.747231633806965e-05, -6.460461787722171e-05, -6.739619325891061e-05, -6.42568749063365e-05, -6.728357578332122e-05, -6.572581320455293e-05, -6.733133575279844e-05, -6.745384605205556e-05, -6.654768580556922e-05, -6.752884945881219e-05, -6.516474446690376e-05, -6.800609459823608e-05, -6.47878614014136e-05, -6.730160658797204e-05, -6.420250070636625e-05, -6.676581343835398e-05, -6.447454426249553e-05, -6.739644425949934e-05, -6.633928104016707e-05, -6.668506011610336e-05, -6.704708770176857e-05, -6.518924517552728e-05, -6.80110716513718e-05, -6.449044290923919e-05, -6.713463098761624e-05, -6.431427908560736e-05, -6.666702370071547e-05, -6.380160055564429e-05, -6.69295226583365e-05, -6.559831844106169e-05, -6.733302905782082e-05, -6.676258268638944e-05, -6.581664753168712e-05, -6.791627178025961e-05, -6.483985086130437e-05, -6.771582429628417e-05, -6.456692771022534e-05, -6.710554331363558e-05, -6.416205680544463e-05, -6.721382973122853e-05, -6.497521331755278e-05, -6.762221774081424e-05, -6.644148745970977e-05, -6.650204706057299e-05, -6.779409446006897e-05, -6.513429971844772e-05, -6.716283035881229e-05, -6.500520220536936e-05, -6.748818593189037e-05, -6.375021526081944e-05, -6.679304519274533e-05, -6.44009832356367e-05, -6.697029619860621e-05, -6.614507717764695e-05, -6.675045380090485e-05, -6.699368958403159e-05, -6.540977419016514e-05, -6.751824094235534e-05, -6.497224203386006e-05, -6.747996187391402e-05, -6.445371747351958e-05, -6.694216412544935e-05, -6.39145549472495e-05, -6.67208337122775e-05, -6.499887641961741e-05, -6.75636406906266e-05, -6.646187561893783e-05, -6.6422353672184e-05, -6.774188283466967e-05, -6.49718493653088e-05, -6.774060340062207e-05, -6.447729538855726e-05, -6.7276329542447e-05, -6.45413468122233e-05, -6.725796598454556e-05, -6.43215545435326e-05, -6.710426281533913e-05, -6.640793922515245e-05, -6.688725807556598e-05, -6.702595030422637e-05, -6.555532275656158e-05, -6.775334049196785e-05, -6.485489689304207e-05, -6.778283710493148e-05, -6.47406497658257e-05, -6.667061103568536e-05, -6.71178176816977e-05, -6.545036016336727e-05, -6.758648874374465e-05, -6.648186107488955e-05, -6.564351224820166e-05, -6.726344507999936e-05, -6.562770441403993e-05, -6.793015780847218e-05, -6.469220243177453e-05, -6.740767551952607e-05, -6.44720529171589e-05, -6.682838905210087e-05, -6.483406975990464e-05, -6.710332224721377e-05, -6.629467593853179e-05, -6.657765389063085e-05]
  in  "Stream to disk?":bool
  in  "decimating factor":i32
  in  "Input Signals":i16(slide)=2 scale=1.0..20.0
  out "Measure?":u16[](array[numeric])=[2, 1, 2, 2, 2, 1]
  # "*****Customized for 4461 + 4462 cards*****"
  # "Real time Adjustable Values"
  # "Configurations"
  # "The top array index selects which card you are setting the outputs for,and the second index selects which output chanel on that card.\n\nFor Phase&Tc, you must have an array element initialized for each input signal."
  # "Features:\n1, Any number of input and output channels\n2, Each AO outputs an DC+AC signal, DC for sample biasing and AC for OSC. These values can be adjusted in real time.\n3, Synchronous filtering\n\nInstructions:\n1, Array index of AI configuration and AO configuration refers to task.\n2, Array index in Amplifier Settings, Phase$&Tc control , and gains correlates to channel number.\n3, Each 4461 board can have 2 lock-in channels. Syntax for 2 channles, e.g. PXI1Slot2/ai0:1. If you want to use just one, then PXI1Slot2/ai0.\n4, Parameters (especially DC value for sample biasing) can be remotely controlled by clicking \"local\"and \"remote\" button. In real experiments, put golable values (can be found in Lock-in globles.vi) in your VI to control the lock-in and read out.\n5, choose OSC frequencies to be multiple of \nAI Rate/AI Block SIze to have best performance.\n\n-Guanglei 06/23/2011\n\nUpdate:\n1. Allows any number of lockin amplifiers and AO tasks.\n2. Delete the channels from any AI/AO Configuration elements you do not want to use.\n3. Rows (first index) of the OSC Configuration correspond to different AO tasks, while columns (second index) correspond to AO channels in that task. All channels in a given element of the AO Configuration array will go into a single task.\n4. The same number of output channels must go in each AO task.\n5. Make sure a Phase&Tc element and an Amplifier Settings element is set for each AI channel.\n-Joe 12/3/2013"
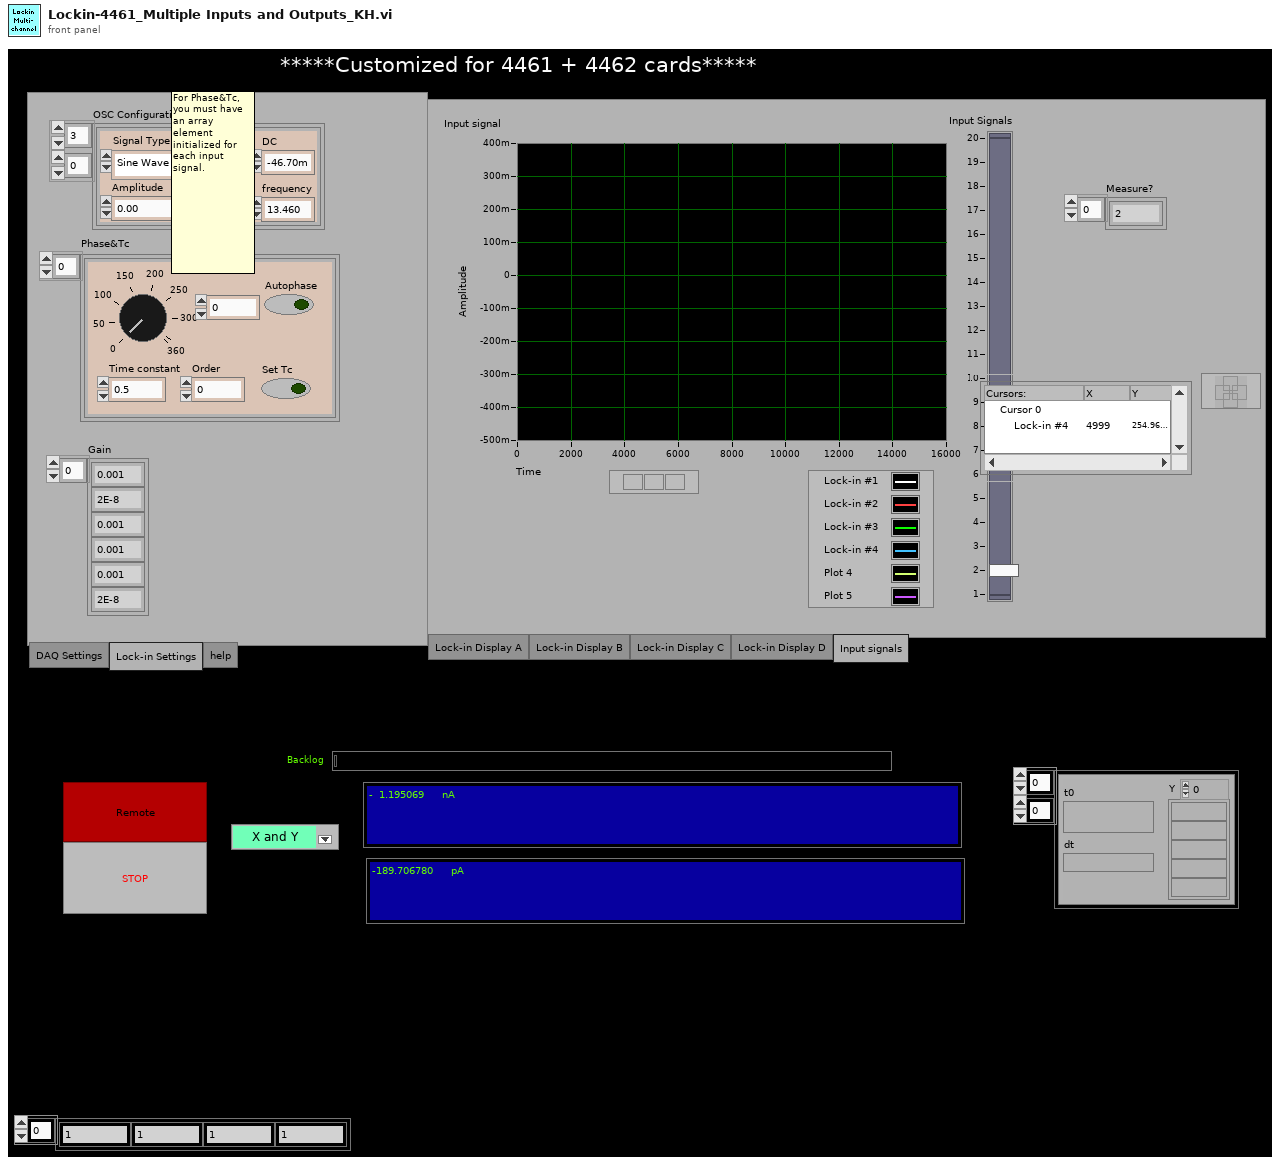
[diagram p1: front panel]
types:
  T1 = enum32{"DAQ Settings", "Lock-in Settings", "help"}
  T2 = cluster{"AI.Coupling":i32, "AI.Max":dbl, "AI.Min":dbl, "Input physical channels":tag}[]
  T3 = cluster{"Output physical channels":tag, "AO. Max":dbl, "AO.Min":dbl}[]
  T4 = cluster{"Signal Type":enum16{"Sine Wave", "Triangle Wave", "Square Wave", "Sawtooth Wave"}, "DC":dbl, "Amplitude":dbl, "frequency":dbl, "Phase":dbl}[][]
  T5 = cluster{"Phase":dbl, "Time constant":dbl, "Set Tc":bool, "Autophase":bool, "Order":dbl}[]
  T6 = enum32{"Lock-in Display A", "Lock-in Display B", "Lock-in Display C", "Lock-in Display D", "Input signals"}
  T7 = cluster{"Signal Type":enum16{"Sine Wave", "Triangle Wave", "Square Wave", "Sawtooth Wave"}, "DC":dbl, "Amplitude":dbl, "frequency":dbl, "Phase":dbl}
  T8 = cluster{"Signal Type":u16, "DC":dbl, "Amplitude":dbl, "frequency":dbl, "Phase":dbl}[][]
  T9 = cluster{"Signal Type":u16, "DC":dbl, "Amplitude":dbl, "frequency":dbl, "Phase":dbl}
  T10 = cluster{"Channel":u16, "Gain":u16, "Shunt Resistor":u16, "Measure":u16}[]
  T11 = cluster{"Ref X":dbl[], "Ref Y":dbl[], "AI Rate":dbl, "AI Block Size":dbl, "Frequency":dbl, "Ref amp":dbl}[]
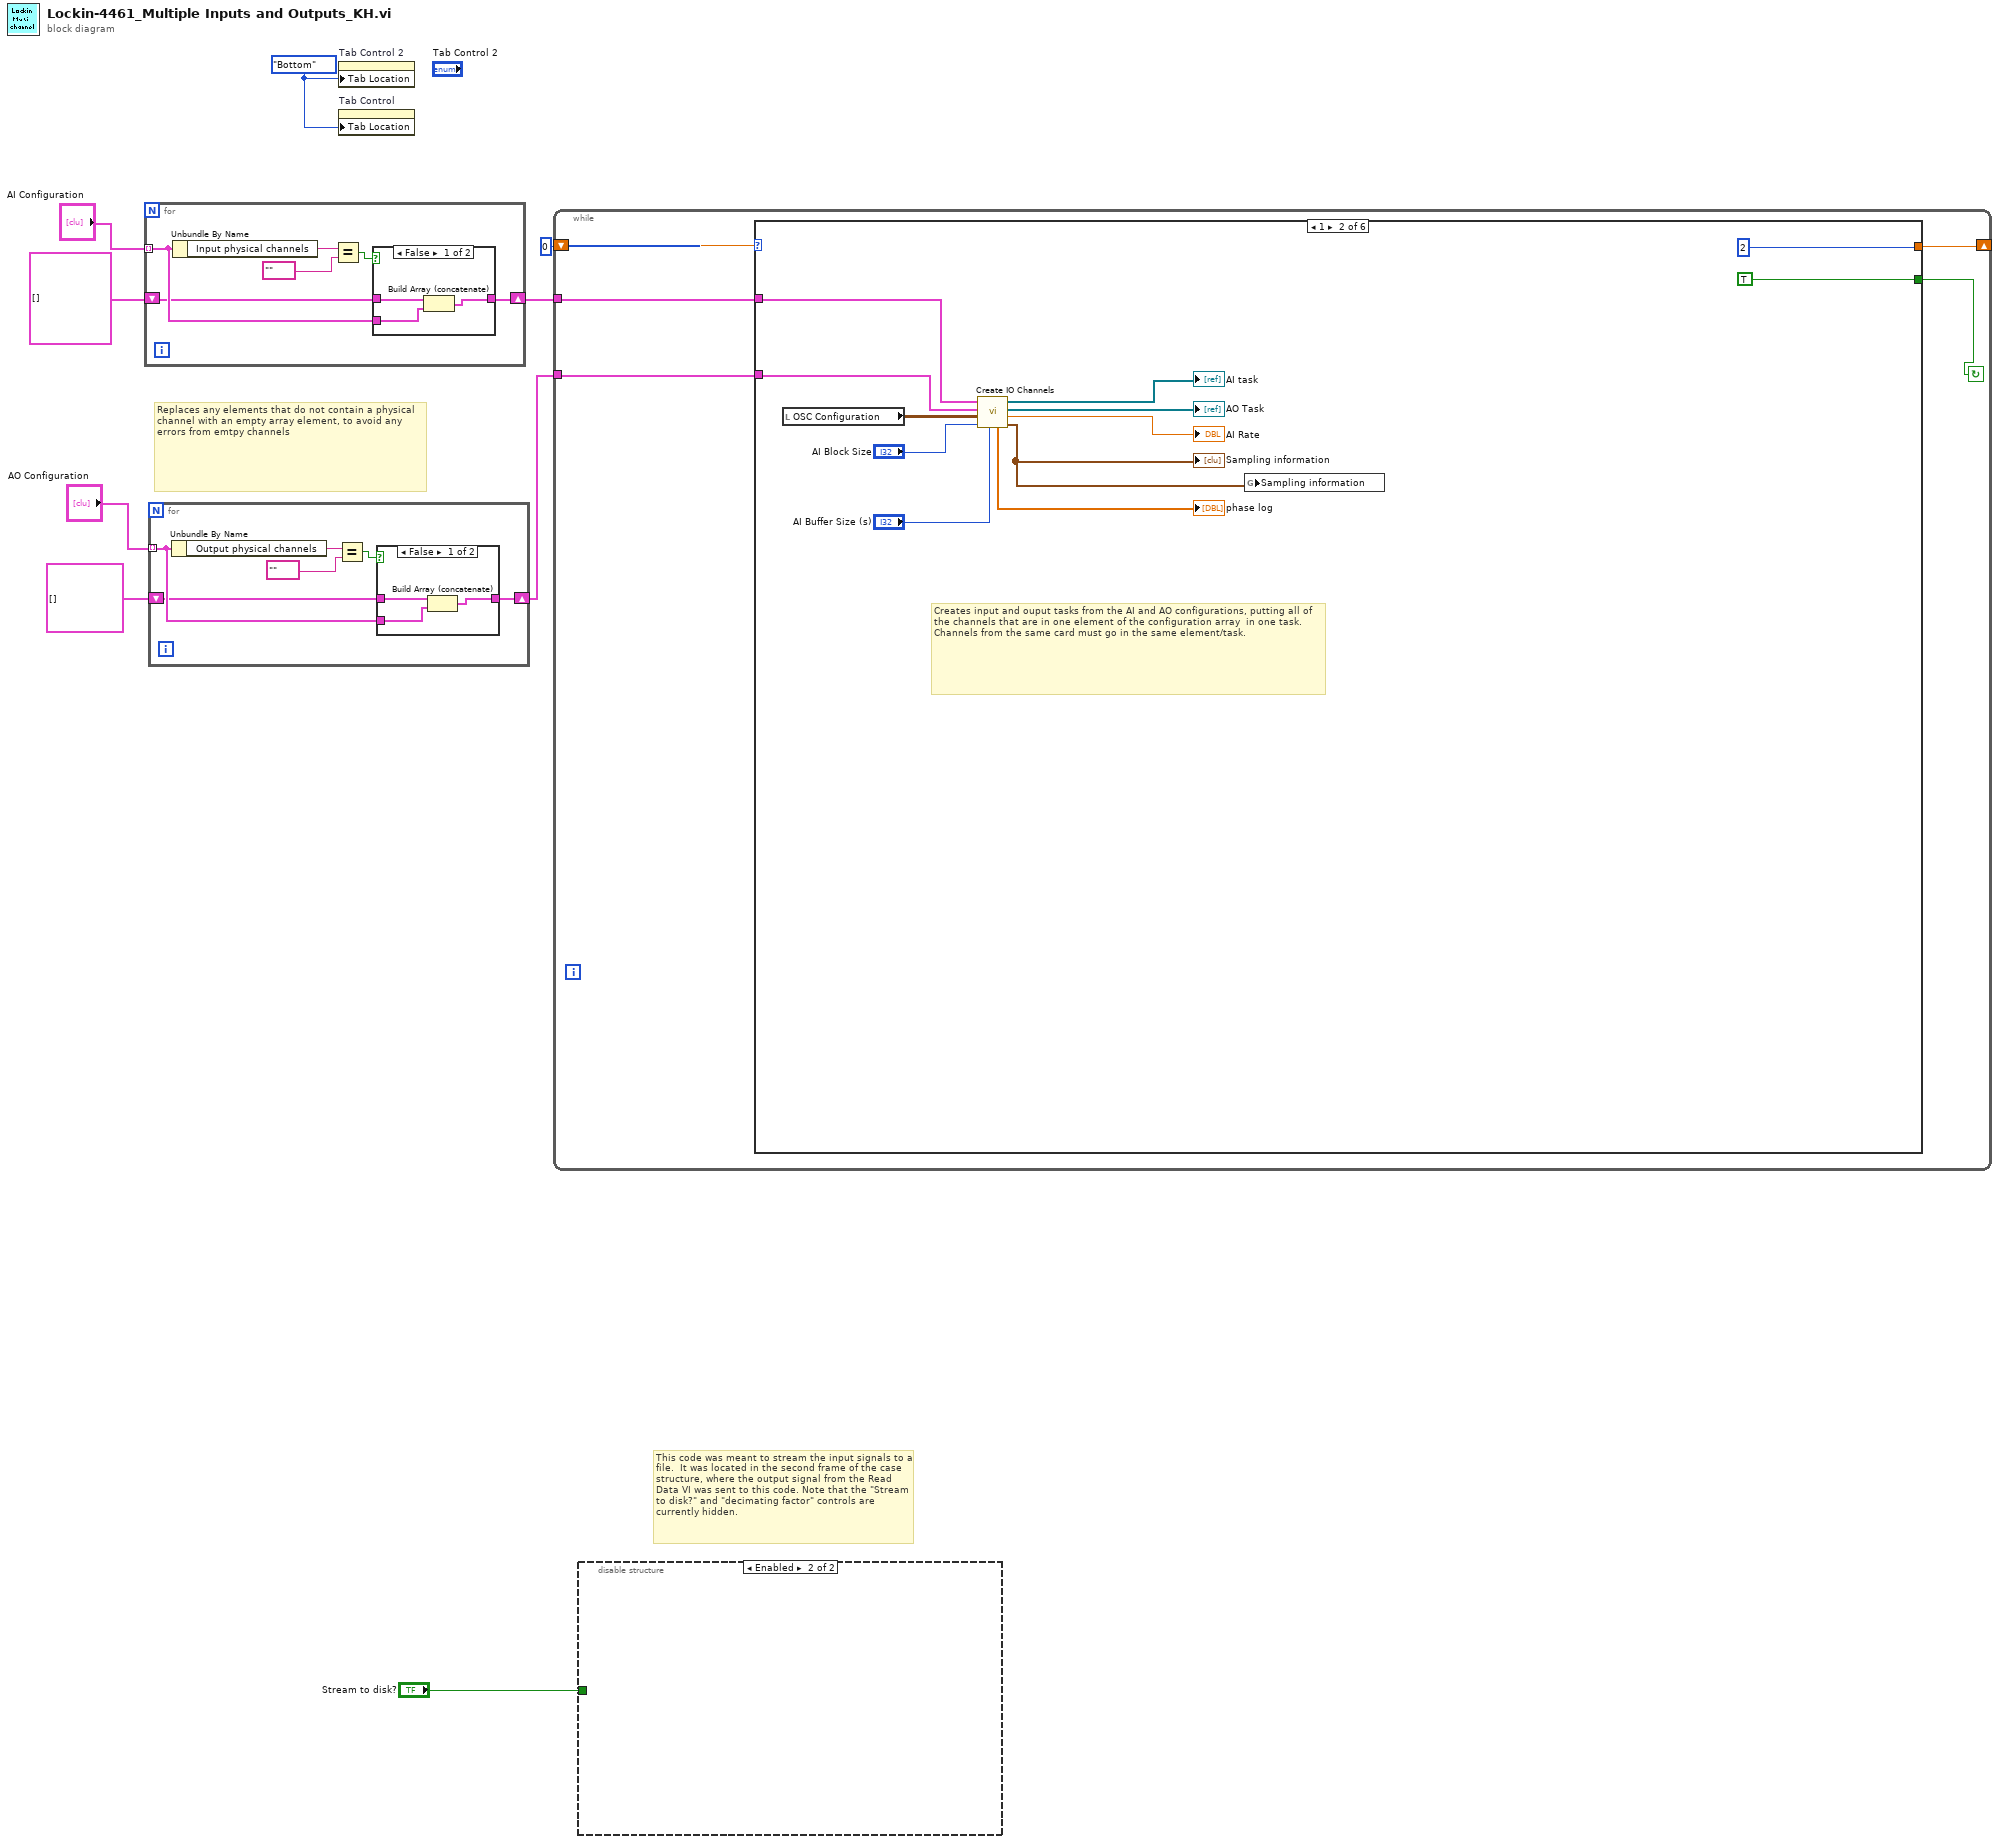
[diagram p0: block diagram]
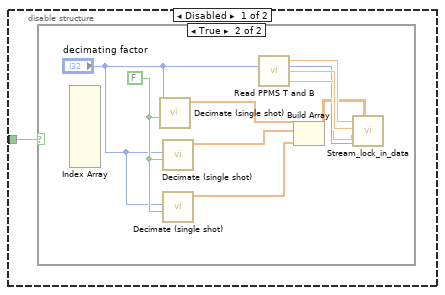
[diagram p2: hidden frame]
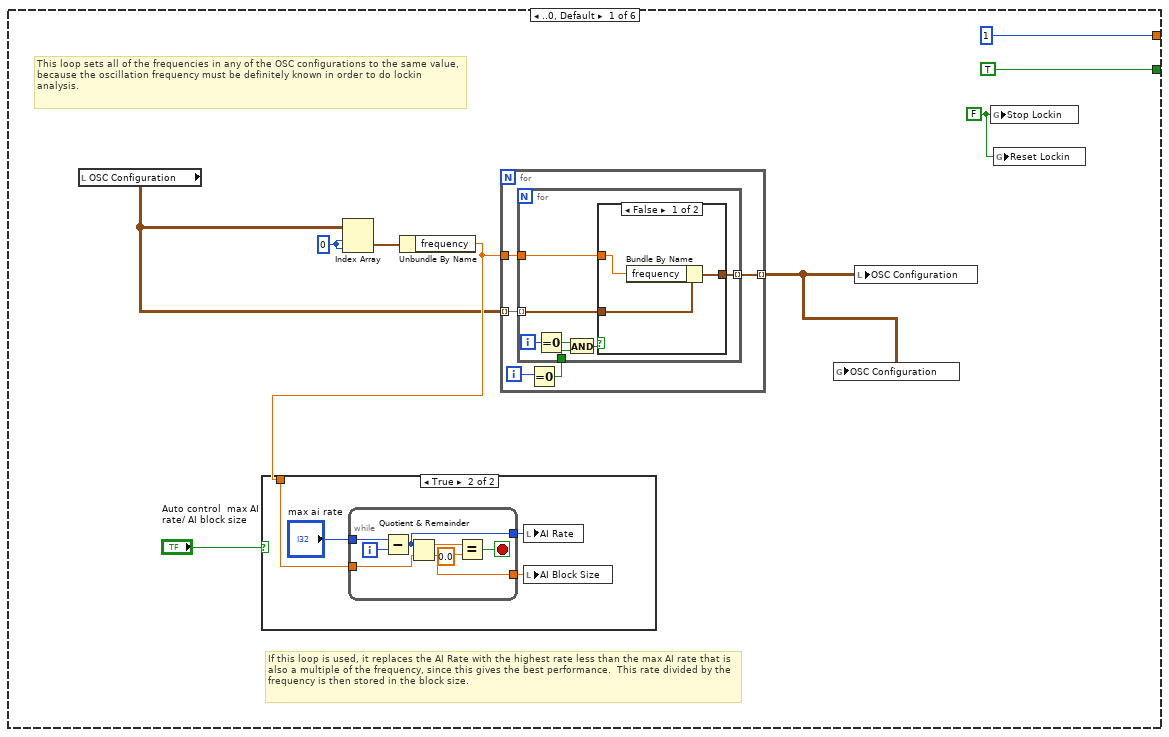
[diagram p6: hidden frame]
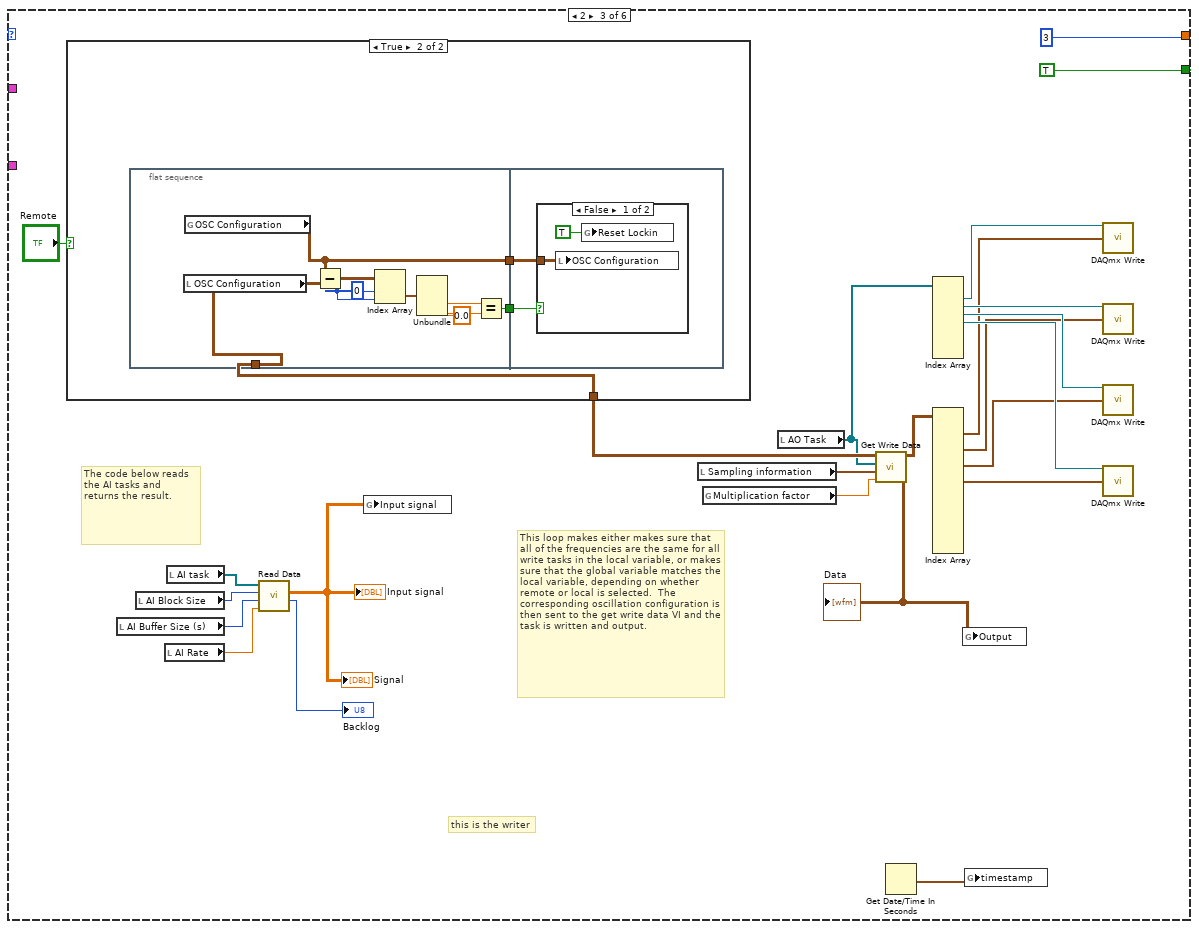
[diagram p9: hidden frame]
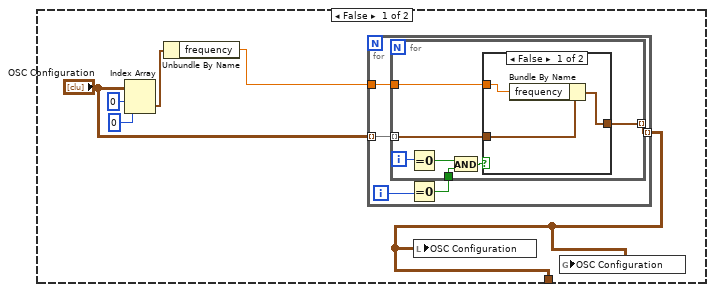
[diagram p10: hidden frame]
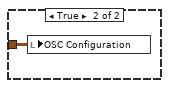
[diagram p12: hidden frame]
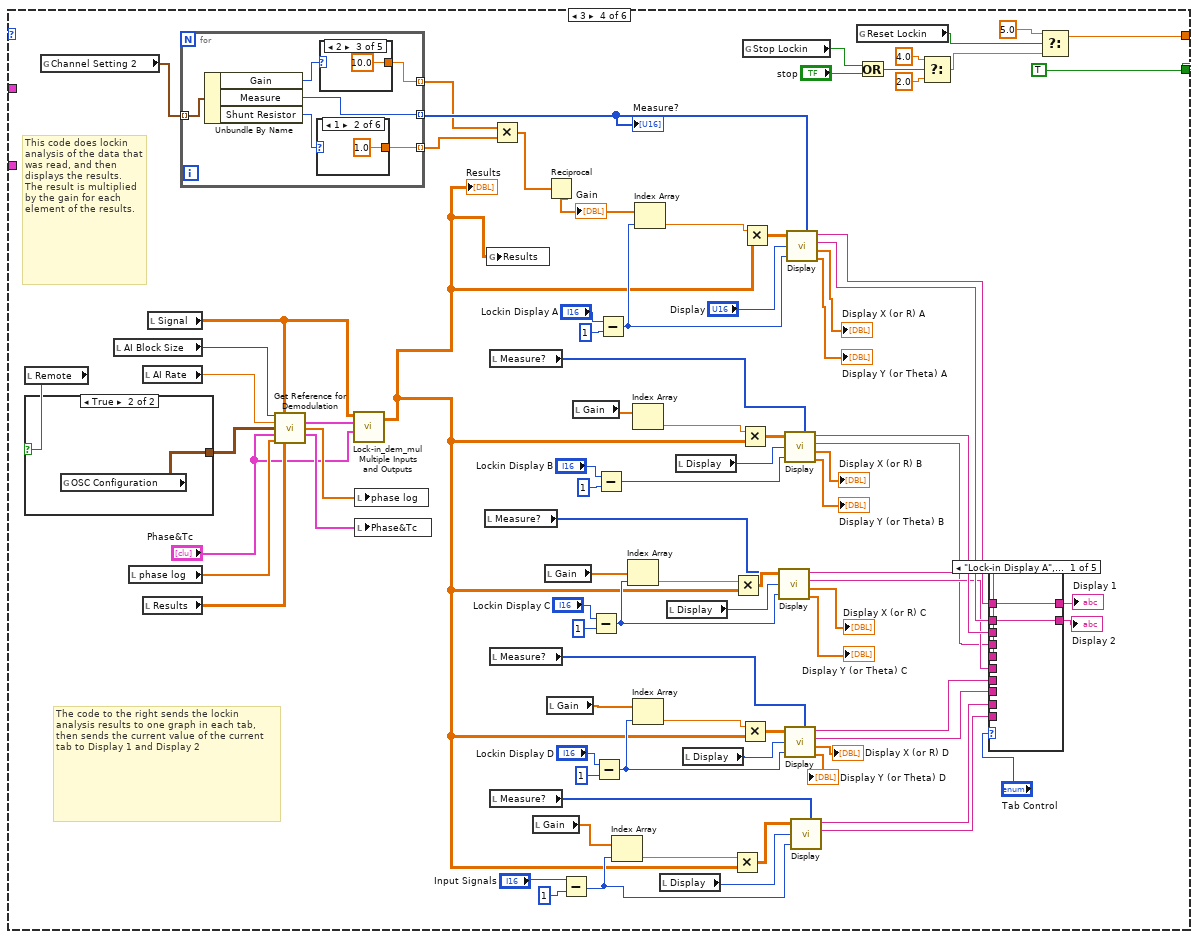
[diagram p13: hidden frame]
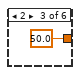
[diagram p15: hidden frame]
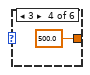
[diagram p16: hidden frame]
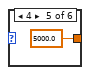
[diagram p17: hidden frame]
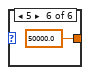
[diagram p18: hidden frame]
diagram:
  w3 = enum32{"Top", "Bottom", "Left", "Right"}."Bottom" ("Tab Location")
  # "This code was meant to stream the input signals to a file.  It was located in the second frame of the case structure, where the output signal from the Read Data VI was sent to this code. Note that the \"Stream to disk?\" and \"decimating factor\" controls are currently hidden."
  # "Replaces any elements that do not contain a physical channel with an empty array element, to avoid any errors from emtpy channels"
  n1 = for {
    tunnel: "AI Configuration" -> [w12] mode=indexing
    shift-right: [w10] -> w9
    shift-left: T2 [] ("AI Configuration") -> [w11]
    n2 = Unbundle By Name(w12) -> ("Input physical channels"=w14:tag)
    n3 = Equal?(x=w14, y=tag "" ("Empty physical channels")) -> (x = y?=w15:bool)
    n4 = case shown="False" w15 {
      tunnel: w12 -> [w17 _]
      tunnel: w11 -> [w18 w19]
      tunnel: [w16 w19] -> w10
      frame False {
        n5 = Build Array (concatenate)(w18, w17) -> (w16:T2)
      }
      frame True {
      }
    }
  }
  n6 = for {
    tunnel: "AO Configuration" -> [w22] mode=indexing
    shift-right: [w20] -> w1
    shift-left: T3 [] ("AO Configuration 2") -> [w21]
    n7 = Unbundle By Name(w22) -> ("Output physical channels"=w24:tag)
    n8 = Equal?(x=w24, y=tag "" ("Empty physical channels")) -> (x = y?=w25:bool)
    n9 = case shown="False" w25 {
      tunnel: w22 -> [w27 _]
      tunnel: w21 -> [w28 w29]
      tunnel: [w26 w29] -> w20
      frame False {
        n10 = Build Array (concatenate)(w28, w27) -> (w26:T3)
      }
      frame True {
      }
    }
  }
  n11 = property on="Tab Control 2" class="TabCtl (strict)"("Tab Location"=w3) -> ()  [unwired: 2 in, 2 out]
  n12 = property on="Tab Control" class="TabCtl (strict)"("Tab Location"=w3) -> ()  [unwired: 2 in, 2 out]
  n13 = while {
    shift-right: [w34] -> _
    shift-left: 0 -> [w33]
    tunnel: w9 -> [w32]
    tunnel: w1 -> [w30]
    stop <- w31 continue-if-true
    n14 = case shown="1" w33 {
      selector: w33 -> [_ _ _ _ w268 _]
      tunnel: [1 2 3 w222 w268 0.0 ("f")] -> w34
      tunnel: w32 -> [_ w78 _ _ _ _]
      tunnel: [TRUE TRUE TRUE TRUE FALSE TRUE] -> w31
      tunnel: w30 -> [_ w77 _ _ _ _]
      frame ..0, Default {
        w38 = 0 ("disabled index (col)")
        w42 = FALSE ("Stop Lockin")
        # "If this loop is used, it replaces the AI Rate with the highest rate less than the max AI rate that is also a multiple of the frequency, since this gives the best performance.  This rate divided by the frequency is then stored in the block size."
        # "This loop sets all of the frequencies in any of the OSC configurations to the same value, because the oscillation frequency must be definitely known in order to do lockin analysis."
        n15 = local read "OSC Configuration"() -> (w36:T4)
        n16 = Index Array(array=w36, index (row)=w38, index (col)=w38) -> (element=w41:T7)
        n17 = Unbundle By Name(w41) -> ("frequency"=w40:dbl)
        n18 = case shown="True" "Auto control  max AI rate/ AI block size" {
          tunnel: w40 -> [_ w62]
          frame False {
          }
          frame True {
            n19 = while {
              tunnel: "max ai rate" -> [w71]
              tunnel: w62 -> [w69]
              tunnel: [w65] -> w61
              tunnel: [w64] -> w60
              i -> [w70]
              stop <- w66 stop-if-true
              n20 = Subtract(x=w71, y=w70) -> (x-y=w64:i32)
              n21 = Quotient & Remainder(x=w64, y=w69) -> (x-y*floor(x/y)=w68:dbl, floor(x/y)=w65:dbl)
              n22 = Equal?(x=w68, y=0.0) -> (x = y?=w66:bool)
            }
            n23 = local write "AI Rate"(w60) -> ()
            n24 = local write "AI Block Size"(w61) -> ()
          }
        }
        n25 = for {
          tunnel: w36 -> [w48] mode=indexing
          tunnel: w40 -> [w47]
          tunnel: [w46] -> w35 mode=indexing
          i -> [w45]
          n26 = Equal To 0?(x=w45) -> (x = 0?=w44:bool)
          n27 = for {
            tunnel: w48 -> [w55] mode=indexing
            tunnel: w47 -> [w54]
            tunnel: [w53] -> w46 mode=indexing
            tunnel: w44 -> [w50]
            i -> [w52]
            n28 = Equal To 0?(x=w52) -> (x = 0?=w51:bool)
            n29 = And(x=w51, y=w50) -> (x .and. y?=w49:bool)
            n30 = case shown="False" w49 {
              tunnel: w55 -> [w58 w59]
              tunnel: w54 -> [w57 _]
              tunnel: [w56 w59] -> w53
              frame False {
                n31 = Bundle By Name(cluster=w58, "frequency"=w57) -> (w56:T7)
              }
              frame True {
              }
            }
          }
        }
        n32 = global write "Lock-in Globles Multiple Inputs and Outputs.vi" "OSC Configuration"(w35) -> ()
        n33 = local write "OSC Configuration"(w35) -> ()
        n34 = global write "Lock-in Globles Multiple Inputs and Outputs used with FGV.vi" "Stop Lockin"(w42) -> ()
        n35 = global write "Lock-in Globles Multiple Inputs and Outputs used with FGV.vi" "Reset Lockin"(w42) -> ()
      }
      frame 1 {
        # "Creates input and ouput tasks from the AI and AO configurations, putting all of the channels that are in one element of the configuration array  in one task.  Channels from the same card must go in the same element/task."
        n36 = local read "OSC Configuration"() -> (w81:T4)
        n37 = call "Create IO Channels.vi"("AI Buffer Size (s)"="AI Buffer Size (s)", "AI Block Size"="AI Block Size", "OSC Configuration"=w81, "AO Configuration"=w77, "AI Configuration"=w78) -> ("Sampling information"=w72:cluster{"Fs":dbl, "#s":dbl}[], "AI Rate"=→"AI Rate":dbl, "AO Task"=→"AO Task":refnum<k21>[], "AI task"=→"AI task":refnum<k21>[], "phase log"=→"phase log":dbl[])  [unwired: 1 in, 1 out]
        "Sampling information" <- w72
        n38 = global write "Lock-in Globles Multiple Inputs and Outputs.vi" "Sampling information"(w72) -> ()
      }
      frame 2 {
        # "this is the writer"
        # "The code below reads the AI tasks and returns the result."
        # "This loop makes either makes sure that all of the frequencies are the same for all write tasks in the local variable, or makes sure that the global variable matches the local variable, depending on whether remote or local is selected.  The corresponding oscillation configuration is then sent to the get write data VI and the task is written and output."
        n39 = case shown="True" "Remote" {
          tunnel: [w107 w131] -> w102
          frame False {
            n40 = Index Array(array="OSC Configuration", index (row)=0, index (col)=0 ("disabled index (col)")) -> (element=w112:T7)
            n41 = Unbundle By Name(w112) -> ("frequency"=w111:dbl)
            n42 = for {
              tunnel: w111 -> [w117]
              tunnel: "OSC Configuration" -> [w116] mode=indexing
              tunnel: [w115] -> w107 mode=indexing
              i -> [w114]
              n43 = Equal To 0?(x=w114) -> (x = 0?=w113:bool)
              n44 = for {
                tunnel: w116 -> [w124] mode=indexing
                tunnel: w117 -> [w123]
                tunnel: [w122] -> w115 mode=indexing
                tunnel: w113 -> [w118]
                i -> [w120]
                n45 = Equal To 0?(x=w120) -> (x = 0?=w119:bool)
                n46 = And(x=w119, y=w118) -> (x .and. y?=w121:bool)
                n47 = case shown="False" w121 {
                  tunnel: w124 -> [w127 w128]
                  tunnel: w123 -> [w126 _]
                  tunnel: [w125 w128] -> w122
                  frame False {
                    n48 = Bundle By Name(cluster=w127, "frequency"=w126) -> (w125:T7)
                  }
                  frame True {
                  }
                }
              }
            }
            n49 = local write "OSC Configuration"(w107) -> ()
            n50 = global write "Lock-in Globles Multiple Inputs and Outputs.vi" "OSC Configuration"(w107) -> ()
          }
          frame True {
            n51 = flat-sequence {
              tunnel: [w135] -> w131
              tunnel: [w132] -> w130
              tunnel: [w134] -> w129
              tunnel: w130 -> [w141]
              tunnel: w129 -> [w140]
              frame #0 {
                w133 = 0 ("index")
                n52 = local read "OSC Configuration"() -> (w135:T4)
                n53 = global read "Lock-in Globles Multiple Inputs and Outputs.vi" "OSC Configuration"() -> (w132:T4)
                n54 = Subtract(x=w132, y=w135) -> (x-y=w139:T8)
                n55 = Index Array(array=w139, index (row)=w133, index (col)=w133) -> (element=w138:T9)
                n56 = Unbundle(w138) -> ("frequency"=w137:dbl)  [unwired: 4 out]
                n57 = Equal?(x=w137, y=0.0) -> (x = y?=w134:bool)
              }
              frame #1 {
                n58 = case shown="False" w140 {
                  tunnel: w141 -> [w143 w144]
                  frame False {
                    n59 = local write "OSC Configuration"(w143) -> ()
                    n60 = global write "Lock-in Globles Multiple Inputs and Outputs used with FGV.vi" "Reset Lockin"(TRUE ("Reset Lockin")) -> ()
                  }
                  frame True {
                    n61 = local write "OSC Configuration"(w144) -> ()
                  }
                }
              }
            }
          }
        }
        n62 = local read "AI Buffer Size (s)"() -> (w97:i32)
        n63 = local read "AI Block Size"() -> (w98:i32)
        n64 = local read "AI Rate"() -> (w96:dbl)
        n65 = local read "AI task"() -> (w99:refnum<k21>[])
        n66 = call "Read Data.vi"("AI Rate"=w96, "AI Buffer Size (s)"=w97, "AI Block Size"=w98, "AI task"=w99) -> ("Backlog"=→"Backlog":u8, "Input Signals"=w85:dbl[][])  [unwired: 6 in]
        "Signal" <- w85
        "Input signal" <- w85
        n67 = global write "Lock-in Globles Multiple Inputs and Outputs.vi" "Input signal"(w85) -> ()
        n68 = local read "Sampling information"() -> (w101:cluster{"Fs":dbl, "#s":dbl}[])
        n69 = global read "Lock-in Globles Multiple Inputs and Outputs used with FGV.vi" "Multiplication factor"() -> (w100:dbl)
        n70 = local read "AO Task"() -> (w94:refnum<k21>[])
        n71 = call "Get Write Data.vi"("Multiplication Factor"=w100, "Sampling information 2"=w101, "AO Task"=w94, "OSC Configuration"=w102) -> ("Data"=w84:waveform(dbl)[][])  [unwired: 7 in]
        "Data" <- w84
        n72 = Get Date/Time In Seconds() -> (seconds since 1Jan1904=w103:timestamp)
        n73 = Index Array(array=w94) -> (element #1=w93:refnum<k21>, element #2=w92:refnum<k21>, element #3=w91:refnum<k21>, element #4=w90:refnum<k21>)  [unwired: 8 in, 4 out]
        n74 = Index Array(array=w84) -> (element #1=w89:waveform(dbl)[], element #2=w88:waveform(dbl)[], element #3=w87:waveform(dbl)[], element #4=w86:waveform(dbl)[])  [unwired: 16 in, 4 out]
        n75 = global write "Lock-in Globles Multiple Inputs and Outputs.vi" "Output"(w84) -> ()
        n76 = global write "Lock-in Globles Multiple Inputs and Outputs used with FGV.vi" "timestamp"(w103) -> ()
        n77 = call-poly <vilib>:"DAQmx Write.vi"("task/channels in"=w93, "data"=w89) -> ()  [unwired: 11 in, 3 out]
        n78 = call-poly <vilib>:"DAQmx Write.vi"("task/channels in"=w92, "data"=w88) -> ()  [unwired: 11 in, 3 out]
        n79 = call-poly <vilib>:"DAQmx Write.vi"("task/channels in"=w91, "data"=w87) -> ()  [unwired: 11 in, 3 out]
        n80 = call-poly <vilib>:"DAQmx Write.vi"("task/channels in"=w90, "data"=w86) -> ()  [unwired: 11 in, 3 out]
      }
      frame 3 {
        # "The code to the right sends the lockin analysis results to one graph in each tab, then sends the current value of the current tab to Display 1 and Display 2"
        # "This code does lockin analysis of the data that was read, and then displays the results.  The result is multiplied by the gain for each element of the results."
        n81 = local read "Remote"() -> (w221:bool)
        n82 = case shown="True" w221 {
          tunnel: [w259 w260] -> w218
          frame False {
            n83 = local read "OSC Configuration"() -> (w259:T4)
          }
          frame True {
            n84 = global read "Lock-in Globles Multiple Inputs and Outputs.vi" "OSC Configuration"() -> (w260:T4)
          }
        }
        n85 = global read "Global Value.vi" "Channel Setting 2"() -> (w152:T10)
        n86 = local read "AI Block Size"() -> (w220:i32)
        n87 = local read "phase log"() -> (w217:dbl[])
        n88 = local read "AI Rate"() -> (w219:dbl)
        n89 = local read "Results"() -> (w216:dbl[][])
        n90 = local read "Signal"() -> (w215:dbl[][])
        n91 = for {
          tunnel: w152 -> [w237] mode=indexing
          tunnel: [w234] -> w151 mode=indexing
          tunnel: [w233] -> w150 mode=indexing
          tunnel: [w235] -> w148 mode=indexing
          n92 = Unbundle By Name(w237) -> ("Gain"=w236:u16, "Measure"=w234:u16, "Shunt Resistor"=w232:u16)
          n93 = case shown="1" w232 {
            selector: w232 -> [w238 _ _ _ _ _]
            tunnel: [w238 1.0 50.0 500.0 5000.0 50000.0] -> w233
            frame 0, Default {
            }
            frame 1 {
            }
            frame 2 {
            }
            frame 3 {
            }
            frame 4 {
            }
            frame 5 {
            }
          }
          n94 = case shown="2" w236 {
            selector: w236 -> [w244 w245 _ _ _]
            tunnel: [w244 w245 10.0 100.0 1000.0] -> w235
            frame 0, Default {
            }
            frame 1 {
            }
            frame 2 {
            }
            frame 3 {
            }
            frame 4 {
            }
          }
        }
        "Measure?" <- w151
        n95 = call "Get Reference for Demodulation.vi"("AI Block Size"=w220, "Signal"=w215, "AI Rate"=w219, "OSC Configuration"=w218, "Phase&Tc"="Phase&Tc", "phase log"=w217, "Results"=w216) -> ("Ref In"=w146:T11, "Phase Log Out"=w214:dbl[], "Phase&Tc Out"=w213:T5)  [unwired: 6 in]
        n96 = call "Lock-in_dem_mul Multiple Inputs and Outputs.vi"("Phase&Tc"="Phase&Tc", "Ref in"=w146, "Signal"=w215) -> ("Demodulation"=w145:dbl[][])  [unwired: 2 in]
        "Results" <- w145
        n97 = local write "phase log"(w214) -> ()
        n98 = local write "Phase&Tc"(w213) -> ()
        n99 = local read "Measure?"() -> (w190:u16[])
        n100 = global write "Lock-in Globles Multiple Inputs and Outputs.vi" "Results"(w145) -> ()
        n101 = local read "Measure?"() -> (w189:u16[])
        n102 = local read "Measure?"() -> (w191:u16[])
        n103 = local read "Measure?"() -> (w159:u16[])
        n104 = Multiply(x=w148, y=w150) -> (x*y=w149:dbl[])
        n105 = local read "Gain"() -> (w160:dbl[])
        n106 = local read "Gain"() -> (w187:dbl[])
        n107 = Reciprocal(x=w149) -> (1/x=w147:dbl[])
        "Gain" <- w147
        n108 = local read "Gain"() -> (w186:dbl[])
        n109 = Subtract(x="Input Signals", y=i16 1) -> (x-y=w154:i16)
        n110 = local read "Gain"() -> (w188:dbl[])
        n111 = Subtract(x="Lockin Display C", y=i16 1) -> (x-y=w196:i16)
        n112 = Subtract(x="Lockin Display D", y=i16 1) -> (x-y=w195:i16)
        n113 = Subtract(x="Lockin Display B", y=i16 1) -> (x-y=w203:i16)
        n114 = Subtract(x="Lockin Display A", y=i16 1) -> (x-y=w204:i16)
        n115 = Index Array(array=w160, index=w154) -> (element=w158:dbl)
        n116 = Index Array(array=w187, index=w196) -> (element=w197:dbl)
        n117 = Index Array(array=w188) -> (element=w202:dbl)  [unwired: 1 in]
        n118 = Index Array(array=w186, index=w195) -> (element=w194:dbl)
        n119 = Index Array(array=w147, index=w204) -> (element=w205:dbl)
        n120 = local read "Display"() -> (w156:u16)
        n121 = local read "Display"() -> (w184:u16)
        n122 = local read "Display"() -> (w185:u16)
        n123 = local read "Display"() -> (w183:u16)
        n124 = Multiply(x=w158, y=w145) -> (x*y=w157:dbl[][])
        n125 = Multiply(x=w197, y=w145) -> (x*y=w198:dbl[][])
        n126 = Multiply(x=w202, y=w145) -> (x*y=w201:dbl[][])
        n127 = Multiply(x=w194, y=w145) -> (x*y=w193:dbl[][])
        n128 = Multiply(x=w205, y=w145) -> (x*y=w206:dbl[][])
        n129 = global read "Lock-in Globles Multiple Inputs and Outputs used with FGV.vi" "Stop Lockin"() -> (w228:bool)
        n130 = call "Display.vi"("Results"=w198, "Display"=w184, "Lock-in #"=w196, "Amplifier Settings"=w190) -> ("Display 1"=w167:string, "Display 2"=w168:string, "Array"=→"Display X (or R) C":dbl[], "Array 2"=→"Display Y (or Theta) C":dbl[])  [unwired: 3 in]
        n131 = call "Display.vi"("Results"=w201, "Display"=w185, "Lock-in #"=w203, "Amplifier Settings"=w189) -> ("Display 1"=w169:string, "Display 2"=w165:string, "Array"=→"Display X (or R) B":dbl[], "Array 2"=→"Display Y (or Theta) B":dbl[])  [unwired: 3 in]
        n132 = call "Display.vi"("Results"=w193, "Display"=w183, "Lock-in #"=w195, "Amplifier Settings"=w191) -> ("Display 1"=w163:string, "Display 2"=w164:string, "Array"=→"Display X (or R) D":dbl[], "Array 2"=→"Display Y (or Theta) D":dbl[])  [unwired: 3 in]
        n133 = call "Display.vi"("Results"=w206, "Display"="Display", "Lock-in #"=w204, "Amplifier Settings"=w151) -> ("Display 1"=w171:string, "Display 2"=w170:string, "Array"=→"Display X (or R) A":dbl[], "Array 2"=→"Display Y (or Theta) A":dbl[])  [unwired: 3 in]
        n134 = call "Display.vi"("Results"=w157, "Display"=w156, "Lock-in #"=w154, "Amplifier Settings"=w159) -> ("Display 1"=w162:string, "Display 2"=w161:string)  [unwired: 3 in, 2 out]
        n135 = global read "Lock-in Globles Multiple Inputs and Outputs used with FGV.vi" "Reset Lockin"() -> (w223:bool)
        n136 = Or(x=w228, y="stop") -> (x .or. y?=w226:bool)
        n137 = Select(t=4.0 ("f"), s=w226, f=2.0) -> (s? t:f=w225:dbl)
        n138 = case shown="\"Lock-in Display A\", Default" "Tab Control" {
          tunnel: w171 -> [w250 _ _ _ _]
          tunnel: [w250 w252 w254 w256 w258] -> w173
          tunnel: w170 -> [w249 _ _ _ _]
          tunnel: [w249 w251 w253 w255 w257] -> w172
          tunnel: w169 -> [_ w252 _ _ _]
          tunnel: w165 -> [_ w251 _ _ _]
          tunnel: w167 -> [_ _ w254 _ _]
          tunnel: w168 -> [_ _ w253 _ _]
          tunnel: w163 -> [_ _ _ w256 _]
          tunnel: w164 -> [_ _ _ w255 _]
          tunnel: w162 -> [_ _ _ _ w258]
          tunnel: w161 -> [_ _ _ _ w257]
          frame "Lock-in Display A", Default {
          }
          frame "Lock-in Display B" {
          }
          frame "Lock-in Display C" {
          }
          frame "Lock-in Display D" {
          }
          frame "Input signals" {
          }
        }
        "Display 2" <- w172
        "Display 1" <- w173
        n139 = Select(t=5.0, s=w223, f=w225) -> (s? t:f=w222:dbl)
      }
      frame 4 {
        # "This code stops the AI/AO Tasks, erases them, and ends program execution."
        n140 = local read "AO Task"() -> (w265:refnum<k21>[])
        n141 = local read "AI task"() -> (w267:refnum<k21>[])
        n142 = flat-sequence {
          tunnel: w267 -> [w279]
          tunnel: [w278] -> w266
          tunnel: w265 -> [w278]
          tunnel: [w277] -> w264
          tunnel: w266 -> [w285]
          tunnel: w264 -> [w284]
          tunnel: [w284] -> w263
          tunnel: [w283] -> w262
          frame #0 {
            n143 = for {
              tunnel: w279 -> [w282] mode=indexing
              tunnel: [w280] -> w277 mode=indexing
              n144 = call <vilib>:"DAQmx Stop Task.vi"("task/channels in"=w282) -> ("task out"=w280:refnum<k21>)  [unwired: 13 in, 1 out]
              n145 = Wait (ms)(milliseconds to wait=u32 50) -> ()  [unwired: 1 out]
            }
          }
          frame #1 {
            n146 = for {
              tunnel: w285 -> [w288] mode=indexing
              tunnel: [w286] -> w283 mode=indexing
              n147 = call <vilib>:"DAQmx Stop Task.vi"("task/channels in"=w288) -> ("task out"=w286:refnum<k21>)  [unwired: 13 in, 1 out]
              n148 = Wait (ms)(milliseconds to wait=u32 50) -> ()  [unwired: 1 out]
            }
          }
        }
        n149 = flat-sequence {
          tunnel: w263 -> [w271]
          tunnel: w262 -> [w270]
          tunnel: [w270] -> w261
          tunnel: w261 -> [w274]
          frame #0 {
            n150 = for {
              tunnel: w271 -> [w273] mode=indexing
              n151 = Wait (ms)(milliseconds to wait=u32 50) -> ()  [unwired: 1 out]
              n152 = call <vilib>:"DAQmx Clear Task.vi"("task in"=w273) -> ()  [unwired: 14 in, 1 out]
            }
          }
          frame #1 {
            n153 = for {
              tunnel: w274 -> [w276] mode=indexing
              n154 = call <vilib>:"DAQmx Clear Task.vi"("task in"=w276) -> ()  [unwired: 14 in, 1 out]
              n155 = Wait (ms)(milliseconds to wait=u32 50) -> ()  [unwired: 1 out]
            }
          }
        }
      }
      frame 5 {
        # "This code stops AI/AO tasks, deletes them, and restarts program execution."
        n156 = local read "AO Task"() -> (w292:refnum<k21>[])
        n157 = local read "AI task"() -> (w293:refnum<k21>[])
        n158 = flat-sequence {
          tunnel: w293 -> [w300]
          tunnel: [w299] -> w295
          tunnel: w292 -> [w299]
          tunnel: [w298] -> w294
          tunnel: w295 -> [w306]
          tunnel: w294 -> [w305]
          tunnel: [w305] -> w291
          tunnel: [w304] -> w290
          tunnel: w291 -> [w310]
          tunnel: w290 -> [w311]
          tunnel: [w311] -> w289
          tunnel: w289 -> [w314]
          frame #0 {
            n159 = for {
              tunnel: w300 -> [w303] mode=indexing
              tunnel: [w301] -> w298 mode=indexing
              n160 = Wait (ms)(milliseconds to wait=u32 50) -> ()  [unwired: 1 out]
              n161 = call <vilib>:"DAQmx Stop Task.vi"("task/channels in"=w303) -> ("task out"=w301:refnum<k21>)  [unwired: 13 in, 1 out]
            }
          }
          frame #1 {
            n162 = for {
              tunnel: w306 -> [w309] mode=indexing
              tunnel: [w307] -> w304 mode=indexing
              n163 = Wait (ms)(milliseconds to wait=u32 50) -> ()  [unwired: 1 out]
              n164 = call <vilib>:"DAQmx Stop Task.vi"("task/channels in"=w309) -> ("task out"=w307:refnum<k21>)  [unwired: 13 in, 1 out]
            }
          }
          frame #2 {
            n165 = for {
              tunnel: w310 -> [w313] mode=indexing
              n166 = call <vilib>:"DAQmx Clear Task.vi"("task in"=w313) -> ()  [unwired: 14 in, 1 out]
              n167 = Wait (ms)(milliseconds to wait=u32 50) -> ()  [unwired: 1 out]
            }
          }
          frame #3 {
            n168 = for {
              tunnel: w314 -> [w316] mode=indexing
              n169 = call <vilib>:"DAQmx Clear Task.vi"("task in"=w316) -> ()  [unwired: 14 in, 1 out]
              n170 = Wait (ms)(milliseconds to wait=u32 50) -> ()  [unwired: 1 out]
            }
          }
        }
      }
    }
  }
  n171 = disable-structure shown="Enabled" {
    disable-tunnel: "Stream to disk?" -> [w317 _]
    frame Disabled {
      n172 = case shown="True" w317 {
        frame False {
        }
        frame True {
          w326 = FALSE ("averaging")
          n173 = Index Array() -> ()  [unwired: 9 in, 4 out]
          n174 = call-poly <vilib>:"Decimate (single shot).vi"("averaging"=w326, "decimating factor"="decimating factor") -> ("Decimated Array"=w325:dbl[])  [unwired: 8 in, 1 out]
          n175 = call-poly <vilib>:"Decimate (single shot).vi"("averaging"=w326, "decimating factor"="decimating factor") -> ("Decimated Array"=w324:dbl[])  [unwired: 8 in, 1 out]
          n176 = call-poly <vilib>:"Decimate (single shot).vi"("averaging"=w326, "decimating factor"="decimating factor") -> ("Decimated Array"=w323:dbl[])  [unwired: 8 in, 1 out]
          n177 = call <userlib>:"Read PPMS T and B.vi"() -> ("Field"=w320:dbl, "Temperature"=w321:dbl, "Time"=w322:dbl)  [unwired: 3 in]
          n178 = Build Array(w325, w324, w323) -> (w319:dbl[][])
          n179 = call "Stream_lock_in_data.vi"("Input signal 2"=w319, "decimating factor"="decimating factor", "Field"=w320, "Temperature"=w321, "Time"=w322) -> ()  [unwired: 4 in]
        }
      }
    }
    frame Enabled {
    }
  }
